vi "BRig_RT_panel_Laser1_v1,11.vi"(7 "input_setValues":bool, 9 "input_dataExp":u16[](array[numeric]), 11 "input_dataLC":u16[](array[numeric])) -> (1 "output_dataExp":u16[](array[numeric]), 3 "output_dataLC":u16[](array[numeric]))   [LabVIEW 2014]
panel:
  in  "LC_Sel_nRew2":u16
  in  "LC_Sel_nRew1":u16
  in  "LC_Cue2_nRew2":u16
  in  "LC_Cue2_nRew1":u16
  in  "LC_Cue_nRew2":u16
  in  "LC_Cue_nRew1":u16
  in  "LC_ENL2_nRew2":u16
  in  "LC_ENL2_nRew1":u16
  in  "LC_ENL_nRew2":u16
  in  "LC_ENL_nRew1":u16
  in  "LC_Cue2_PostR_Count":u16
  in  "LC_Cue2_PostR_delayOpt":bool
  in  "LC_Cue2_PostR_Probability":u16
  in  "LC_Cue2_PostR_Block":u16(slide) max=2 step=1 scale=0.0..2.0
  in  "LC_Cue2_PostR_OnOff":bool
  in  "LC_Cue2_PostR_Tdelay":u16
  in  "LC_ENL2_PostR_delayOpt":bool
  in  "LC_ENL2_PostR_Count":u16
  in  "LC_ENL2_PostR_Probability":u16 max=100 step=1
  in  "LC_ENL2_PostR_Block":u16(slide) max=2 step=1 scale=0.0..2.0
  in  "LC_ENL2_PostR_OnOff":bool
  in  "LC_ENL2_PostR_Tdelay":u16
  in  "LC_Cue2_PreR_Count":u16
  in  "LC_Cue2_First_Count":u16
  in  "LC_Cue2_PreR_delayOpt":bool
  in  "LC_ENL2_PreR_delayOpt":bool
  in  "LC_ENL2_PreR_Count":u16
  in  "LC_ENL2_First_Count":u16
  in  "LC_Cue2_First_delayOpt":bool
  in  "LC_ENL2_First_delayOpt":bool
  in  "LC_Cue2_PreR_Probability":u16
  in  "LC_Cue2_PreR_Block":u16(slide) max=2 step=1 scale=0.0..2.0
  in  "LC_Cue2_PreR_OnOff":bool
  in  "LC_Cue2_First_Probability":u16
  in  "LC_Cue2_First_Block":u16(slide) max=2 step=1 scale=0.0..2.0
  in  "LC_Cue2_First_OnOff":bool
  in  "LC_ENL2_PreR_Probability":u16 max=100 step=1
  in  "LC_ENL2_PreR_Block":u16(slide) max=2 step=1 scale=0.0..2.0
  in  "LC_ENL2_PreR_OnOff":bool
  in  "LC_ENL2_First_Probability":u16 max=100 step=1
  in  "LC_ENL2_First_Block":u16(slide) max=2 step=1 scale=0.0..2.0
  in  "LC_Cue2_PreR_Tdelay":u16
  in  "LC_ENL2_PreR_Tdelay":u16
  in  "LC_Cue2_First_Tdelay":u16
  in  "LC_ENL2_First_Tdelay":u16
  in  "LC_ENL2_First_OnOff":bool
  out "LaserPulseTrain":cluster{u16[], u16[]}(graph)
  in  "LED_baseline":bool
  in  "Laser_power_step":dbl
  in  "Laser_power_max":dbl
  in  "Laser_power_min":dbl
  in  "Laser_Tshutter":u16=2
  in  "Laser_Freq":u16=10
  in  "Laser_Tpeak":u16=2
  in  "Laser_T":u16
  in  "LC_Sel_PostR_Count":u16
  in  "LC_Sel_PostR_Probability":u16
  in  "LC_Sel_PostR_Block":u16(slide) max=2 step=1 scale=0.0..2.0
  in  "LC_Sel_PostR_OnOff":bool
  in  "LC_Sel_PostR_Tdelay":u16
  in  "LC_Cue_PostR_Count":u16
  in  "LC_Cue_PostR_delayOpt":bool
  in  "LC_Cue_PostR_Probability":u16
  in  "LC_Cue_PostR_Block":u16(slide) max=2 step=1 scale=0.0..2.0
  in  "LC_Cue_PostR_OnOff":bool
  in  "LC_Cue_PostR_Tdelay":u16
  in  "LC_ENL_PostR_delayOpt":bool
  in  "LC_ENL_PostR_Count":u16
  in  "LC_ENL_PostR_Probability":u16 max=100 step=1
  in  "LC_ENL_PostR_Block":u16(slide) max=2 step=1 scale=0.0..2.0
  in  "LC_ENL_PostR_OnOff":bool
  in  "LC_ENL_PostR_Tdelay":u16
  in  "LC_Sel_PreR_Count":u16
  in  "LC_Sel_First_Count":u16
  in  "LC_Sel_PreR_Probability":u16
  in  "LC_Sel_PreR_Block":u16(slide) max=2 step=1 scale=0.0..2.0
  in  "LC_Sel_PreR_OnOff":bool
  in  "LC_Sel_First_Probability":u16
  in  "LC_Sel_First_Block":u16(slide) max=2 step=1 scale=0.0..2.0
  in  "LC_Sel_First_OnOff":bool
  in  "LC_Sel_PreR_Tdelay":u16
  in  "LC_Sel_First_Tdelay":u16
  in  "LC_Cue_PreR_Count":u16
  in  "LC_Cue_First_Count":u16
  in  "LC_Cue_PreR_delayOpt":bool
  in  "LC_ENL_PreR_delayOpt":bool
  in  "LC_ENL_PreR_Count":u16
  in  "LC_ENL_First_Count":u16
  in  "LC_Cue_First_delayOpt":bool
  in  "LC_ENL_First_delayOpt":bool
  in  "LC_Wrong_Probability":u16
  in  "LC_Wrong_Trial":u16(slide) max=2 step=1 scale=0.0..2.0
  in  "LC_Wrong_Block":u16(slide) max=2 step=1 scale=0.0..2.0
  in  "LC_Wrong_OnOff":bool
  in  "LC_Reward_Probability":u16
  in  "LC_Reward_Trial":u16(slide) max=2 step=1 scale=0.0..2.0
  in  "LC_Reward_Block":u16(slide) max=2 step=1 scale=0.0..2.0
  in  "LC_Reward_OnOff":bool
  in  "LC_Cue_PreR_Probability":u16
  in  "LC_Cue_PreR_Block":u16(slide) max=2 step=1 scale=0.0..2.0
  in  "LC_Cue_PreR_OnOff":bool
  in  "LC_Cue_First_Probability":u16
  in  "LC_Cue_First_Block":u16(slide) max=2 step=1 scale=0.0..2.0
  in  "LC_Cue_First_OnOff":bool
  in  "LC_ENL_PreR_Probability":u16 max=100 step=1
  in  "LC_ENL_PreR_Block":u16(slide) max=2 step=1 scale=0.0..2.0
  in  "LC_ENL_PreR_OnOff":bool
  in  "LC_ENL_First_Probability":u16 max=100 step=1
  in  "LC_ENL_First_Block":u16(slide) max=2 step=1 scale=0.0..2.0
  in  "LC_Wrong_Tdelay":u16
  in  "LC_Cue_PreR_Tdelay":u16
  in  "LC_ENL_PreR_Tdelay":u16
  in  "LC_Reward_Tdelay":u16
  in  "LC_Cue_First_Tdelay":u16
  in  "LC_ENL_First_Tdelay":u16
  in  "LC_ENL_First_OnOff":bool
  # "Laser1 Control\n                               On/Off      Block        Probability [%]   Delay [ms]                              Count"
  # "On/Off      Block        Probability [%]   Delay [ms]                              Count"
  # "Enforced\nNonLick"
  # "Enforced\nNonLick\n     2"
  # "from end"
  # "from end"
  # "First\nTrial"
  # "First\nTrial"
  # "from start"
  # "from start"
  # "from end"
  # "from end"
  # "PreReward\nTrials"
  # "PreReward\nTrials"
  # "from start"
  # "from start"
  # "from end"
  # "from end"
  # "PostReward\nTrials"
  # "PostReward\nTrials"
  # "from start"
  # "from start"
  # "PostReward Option - Trigger after [X1] or [X2] reward\n                                        (0 = ignore this option)"
  # "PostReward Option - Trigger after [X1] or [X2] reward\n                                        (0 = ignore this option)"
  # "Cue"
  # "Cue\n  2"
  # "from end"
  # "from end"
  # "First\nTrial"
  # "First\nTrial"
  # "from start"
  # "from start"
  # "from end"
  # "from end"
  # "PreReward\nTrials"
  # "PreReward\nTrials"
  # "from start"
  # "from start"
  # "from end"
  # "from end"
  # "PostReward\nTrials"
  # "PostReward\nTrials"
  # "from start"
  # "from start"
  # "PostReward Option - Trigger after [X1] or [X2] reward\n                                        (0 = ignore this option)"
  # "PostReward Option - Trigger after [X1] or [X2] reward\n                                        (0 = ignore this option)"
  # "Selection"
  # "from start"
  # "First\nTrial"
  # "from start"
  # "PreReward\nTrials"
  # "from start"
  # "PostReward\nTrials"
  # "PostReward Option - Trigger after [X1] or [X2] reward\n                                        (0 = ignore this option)"
  # "Laser1 Parameters"
  # "Laser1 Response\n           On/Off      Block           Trial     Probability %  Delay [ms]"
  # "Frequency\n[Hz]"
  # "Selection\nReward"
  # "Timing [ms]\n Duration     Peak Width   Shutter"
  # "Selection\nWrong"
  # "Laser Power [V]\nMin          Max              Step"
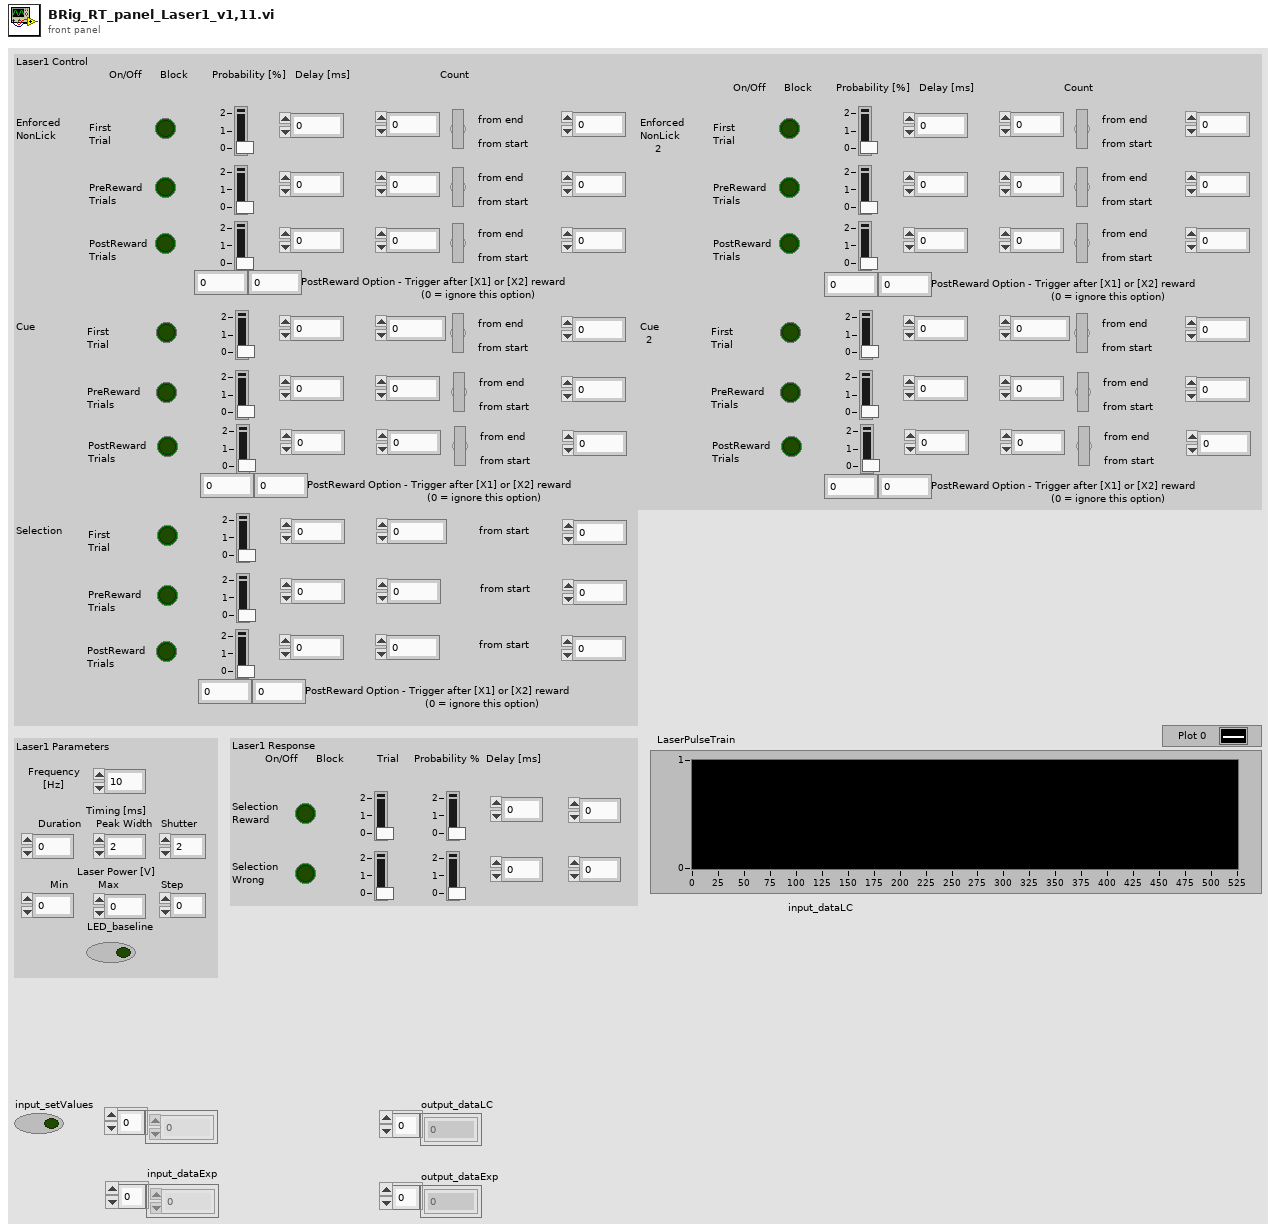
[diagram p1: front panel]
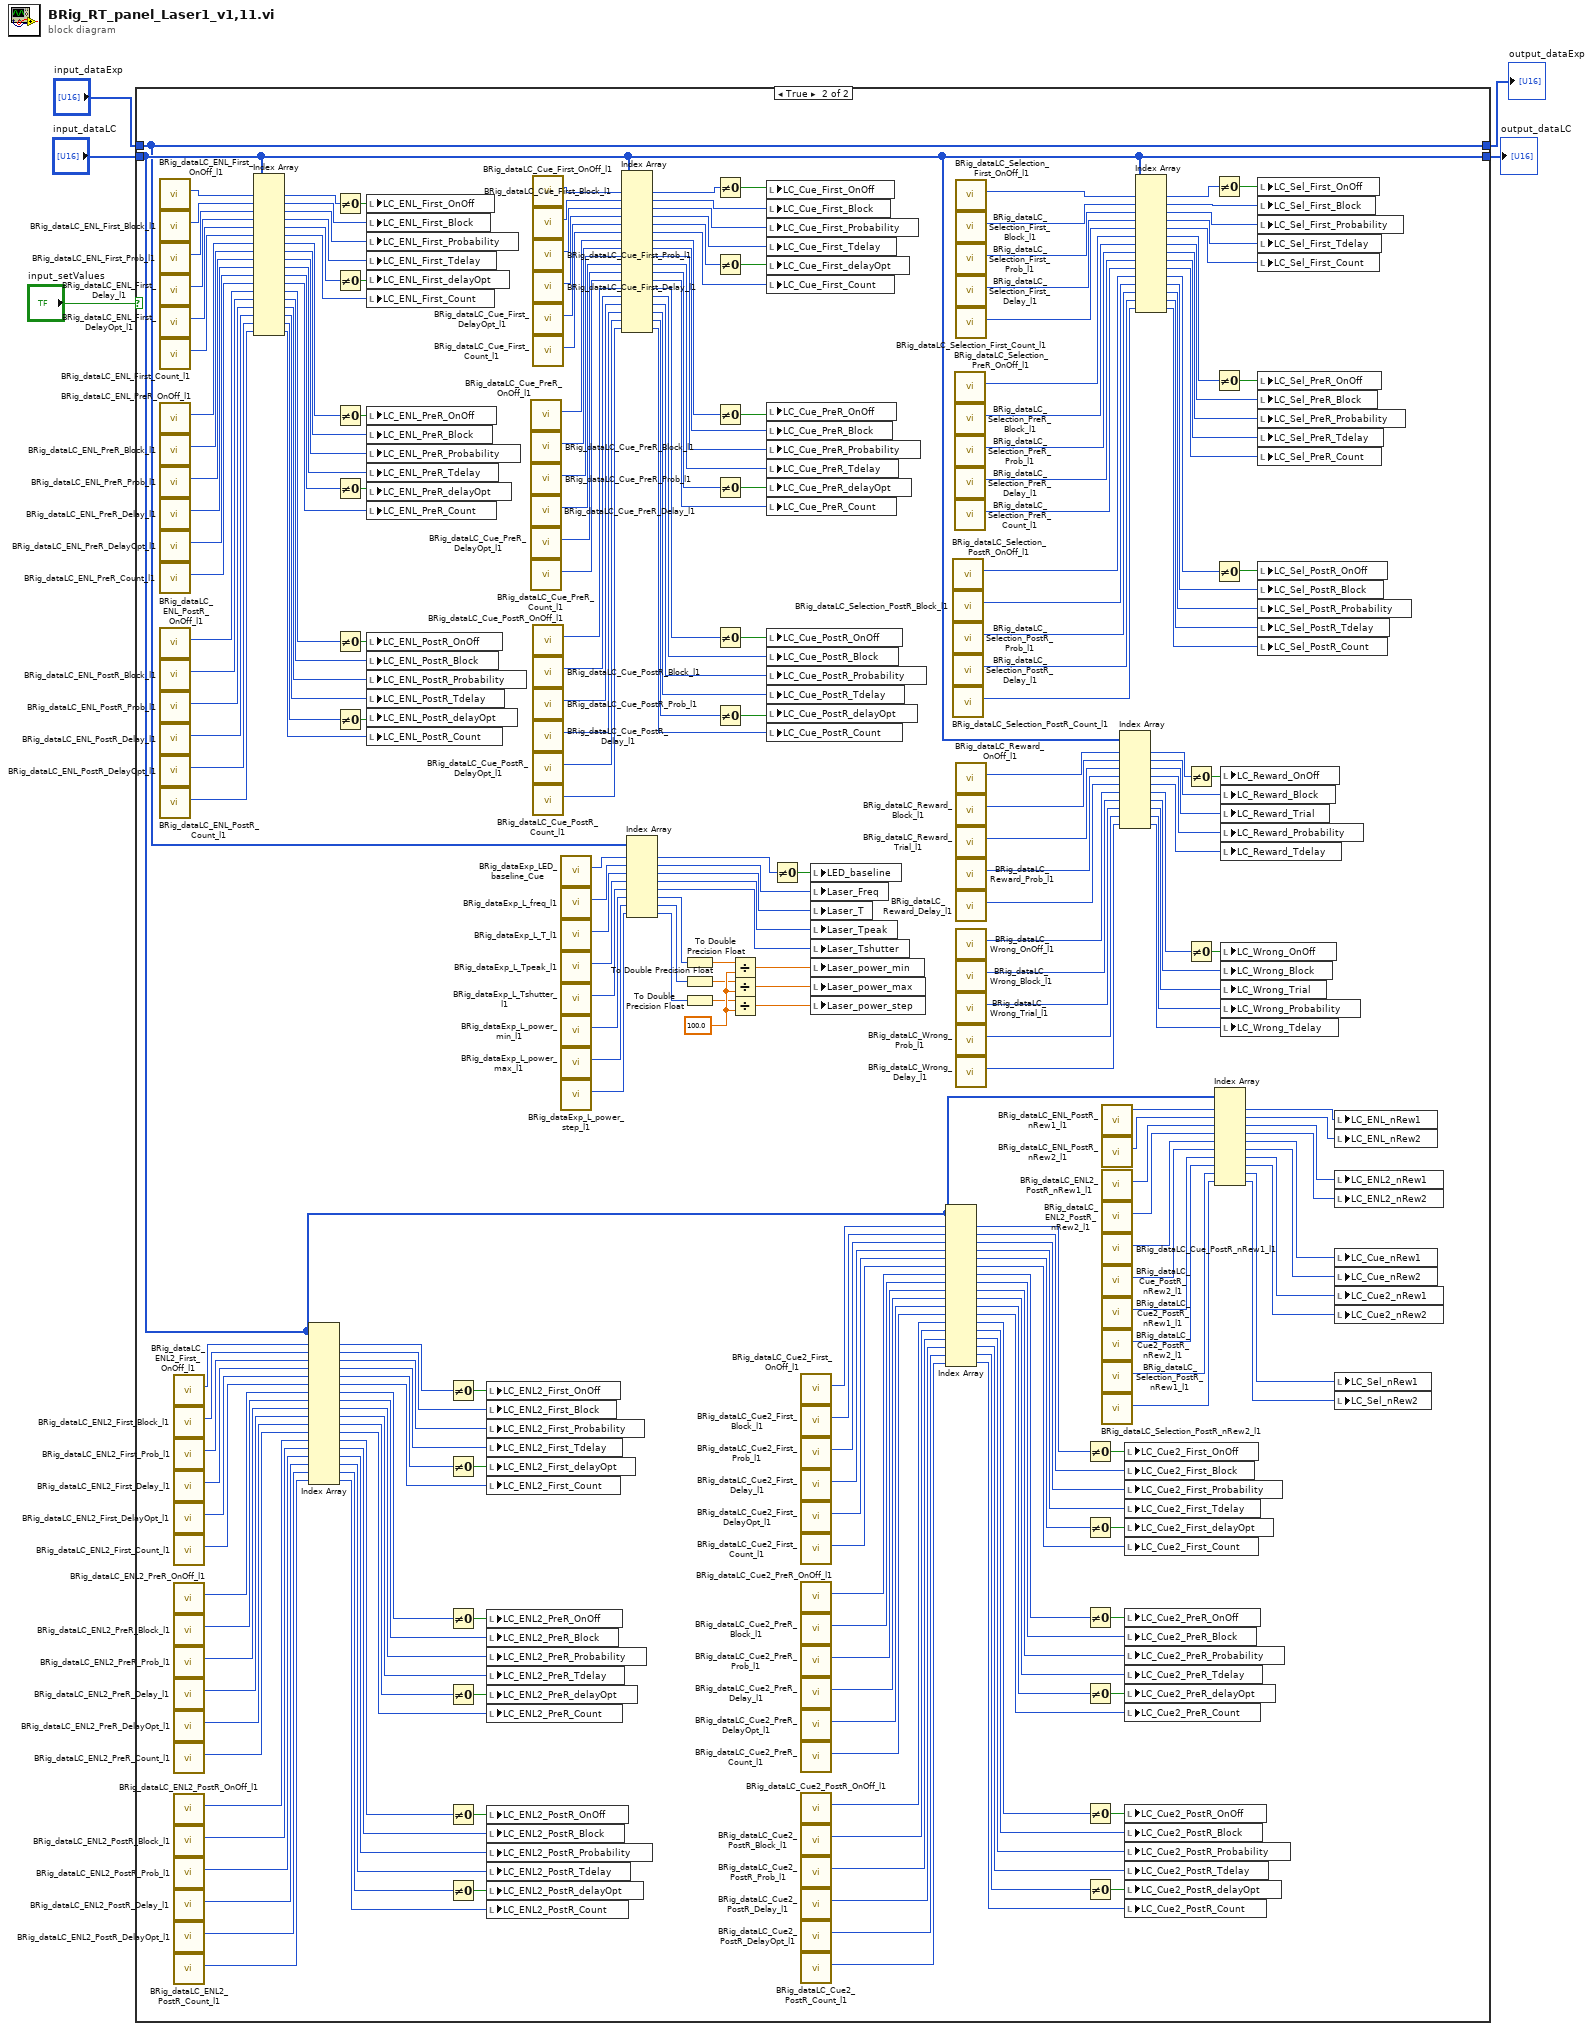
[diagram p0: block diagram]
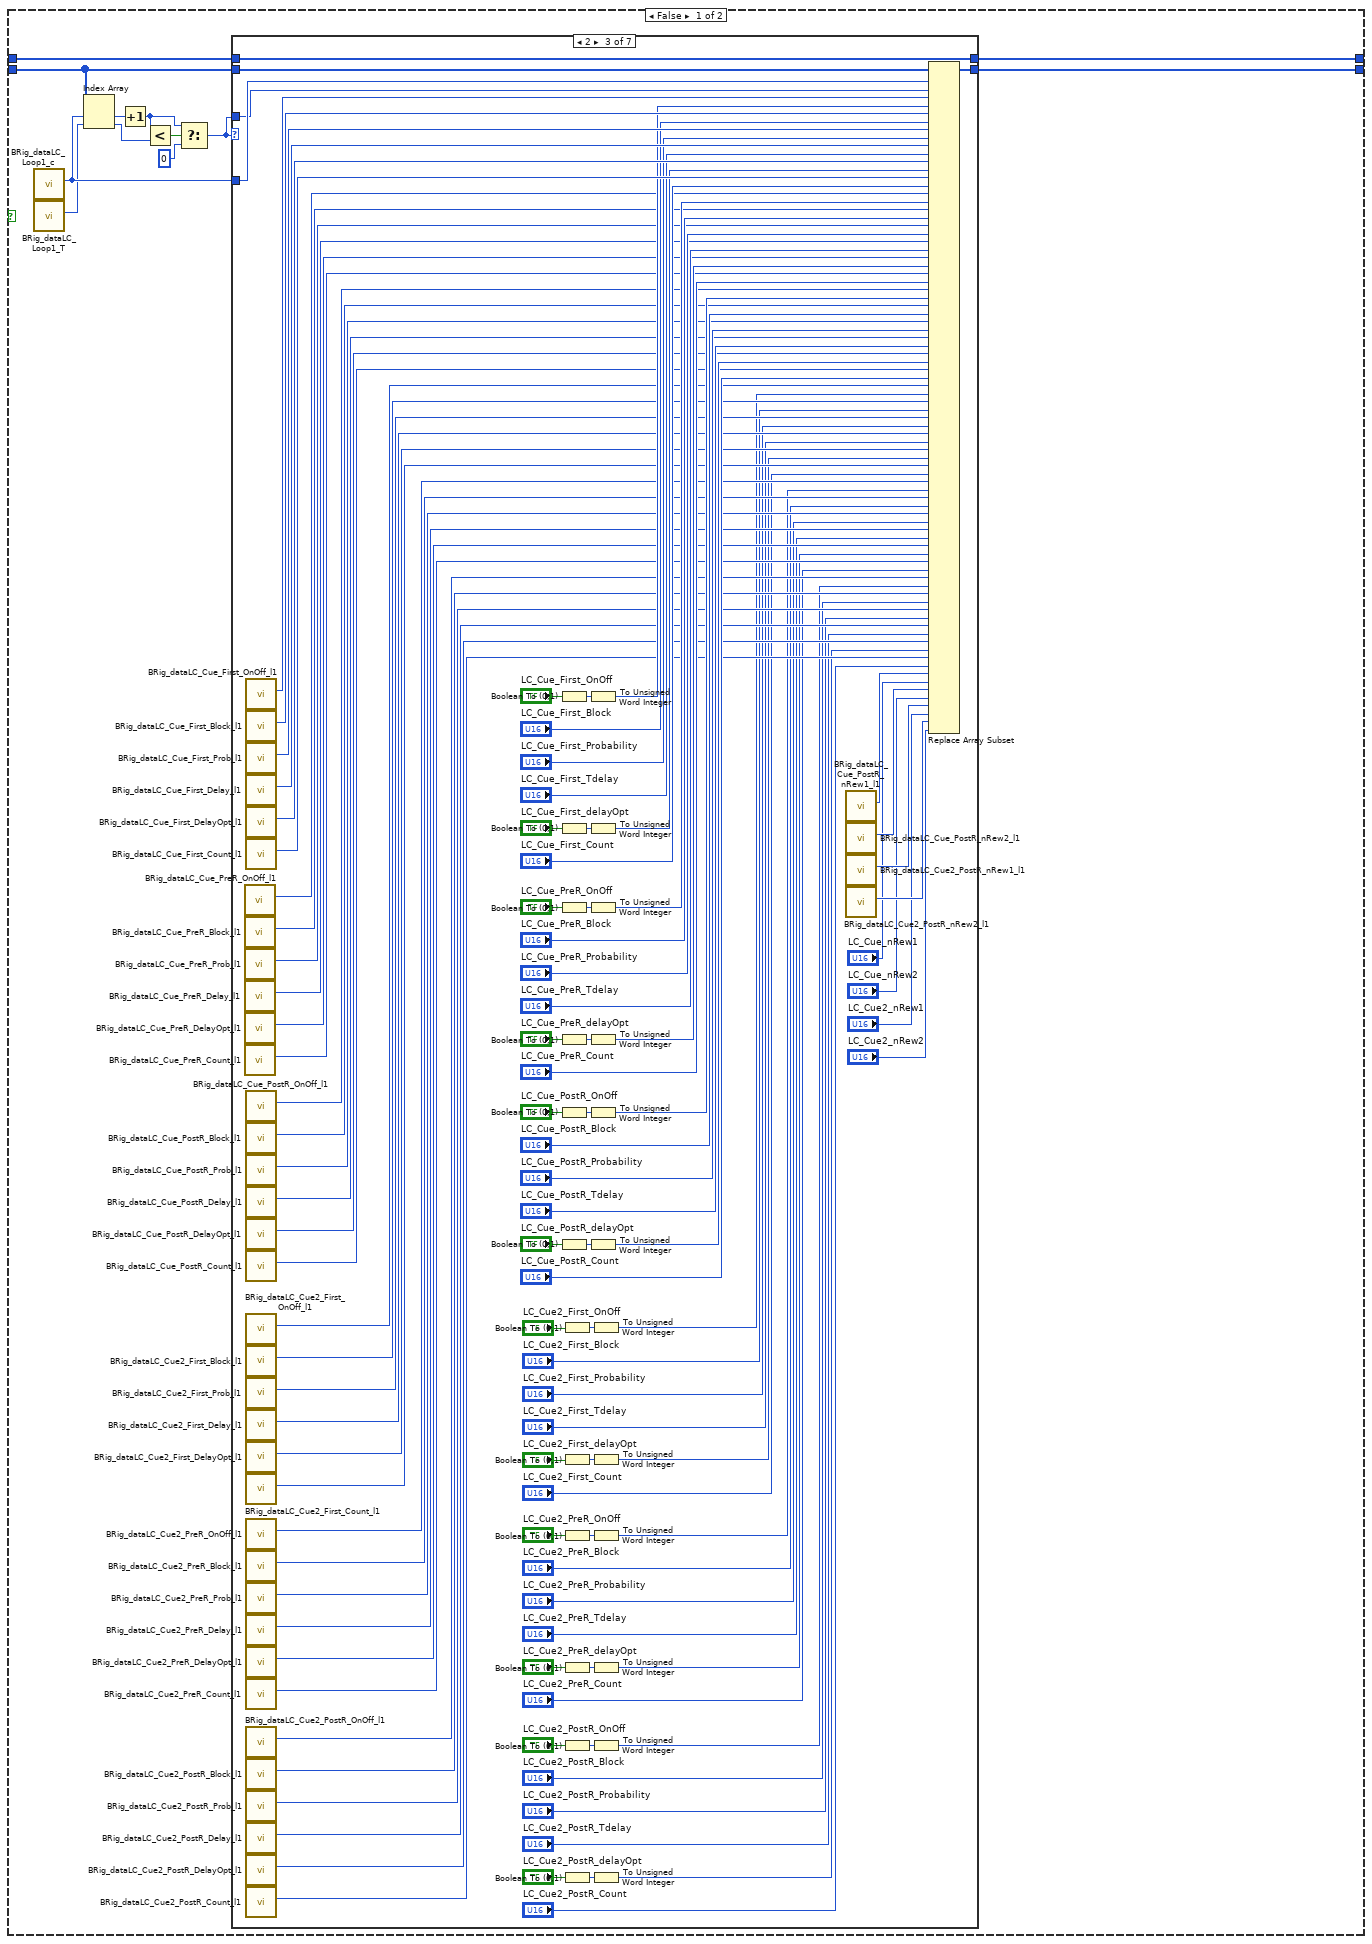
[diagram p2: hidden frame]
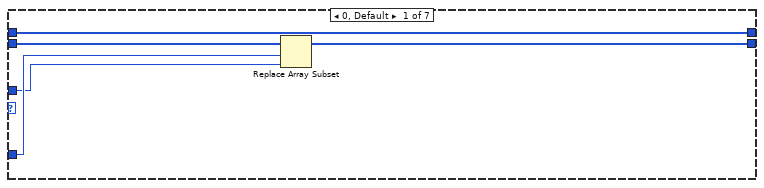
[diagram p3: hidden frame]
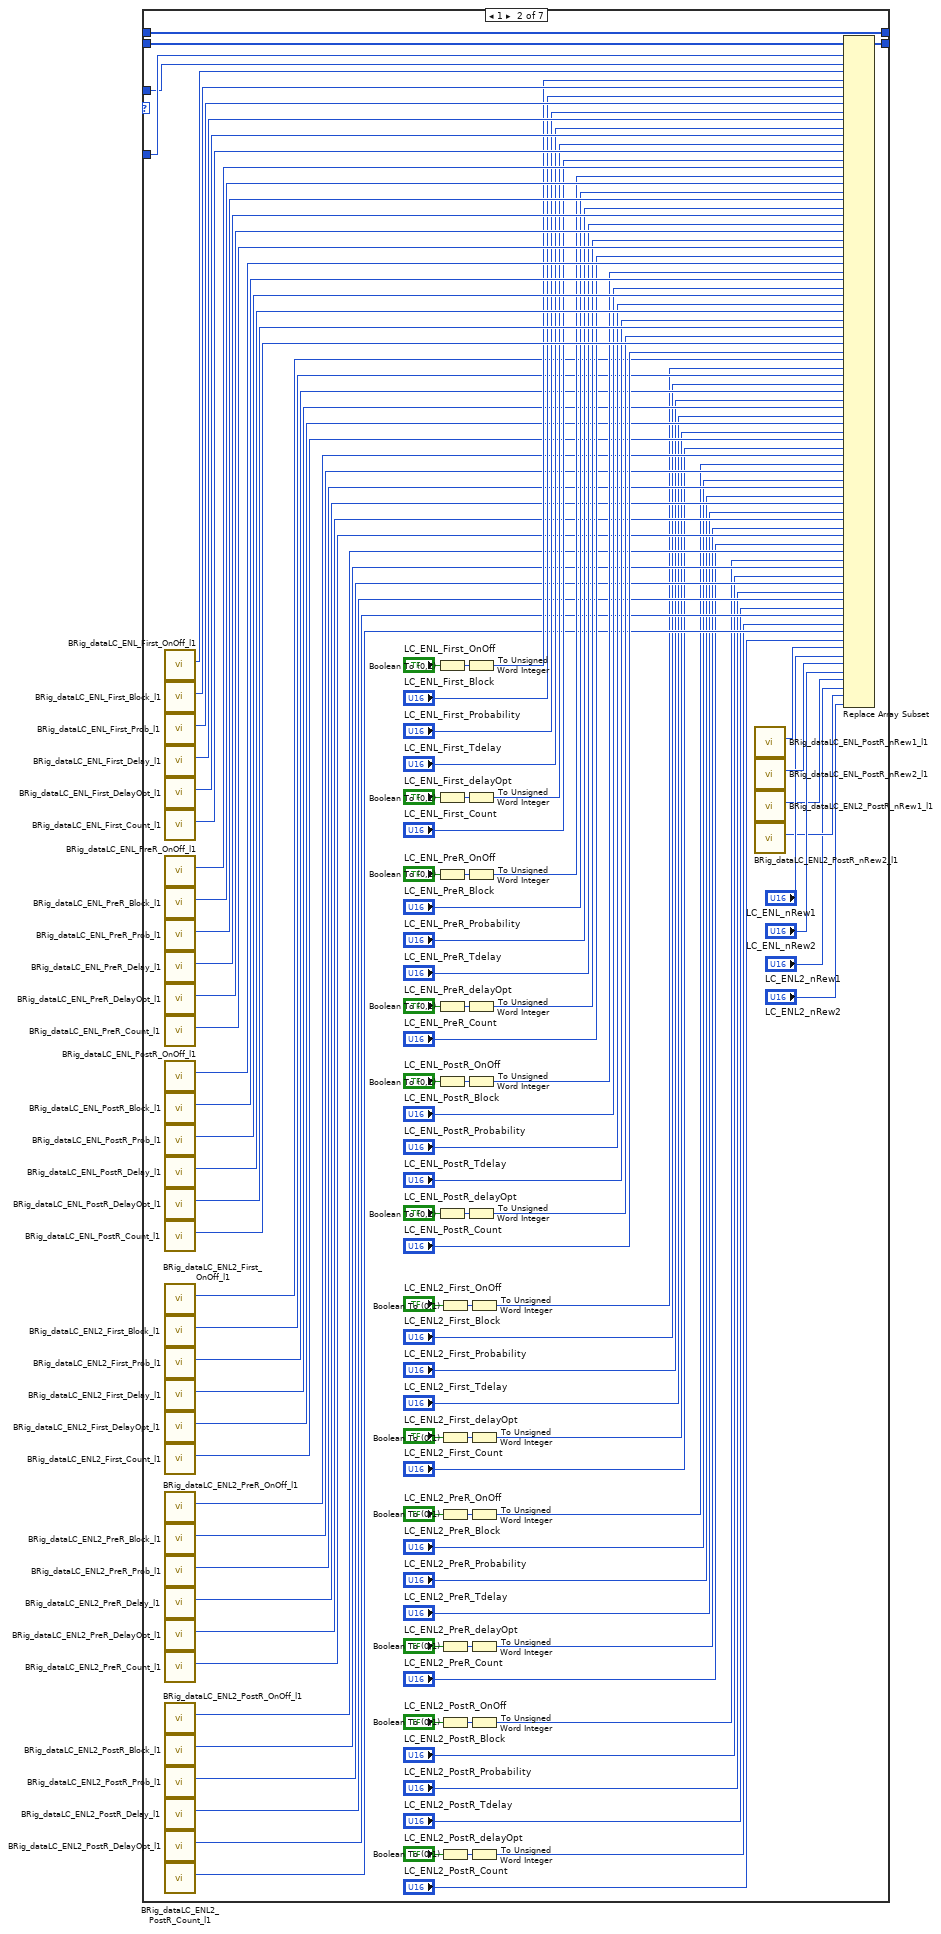
[diagram p4: hidden frame]
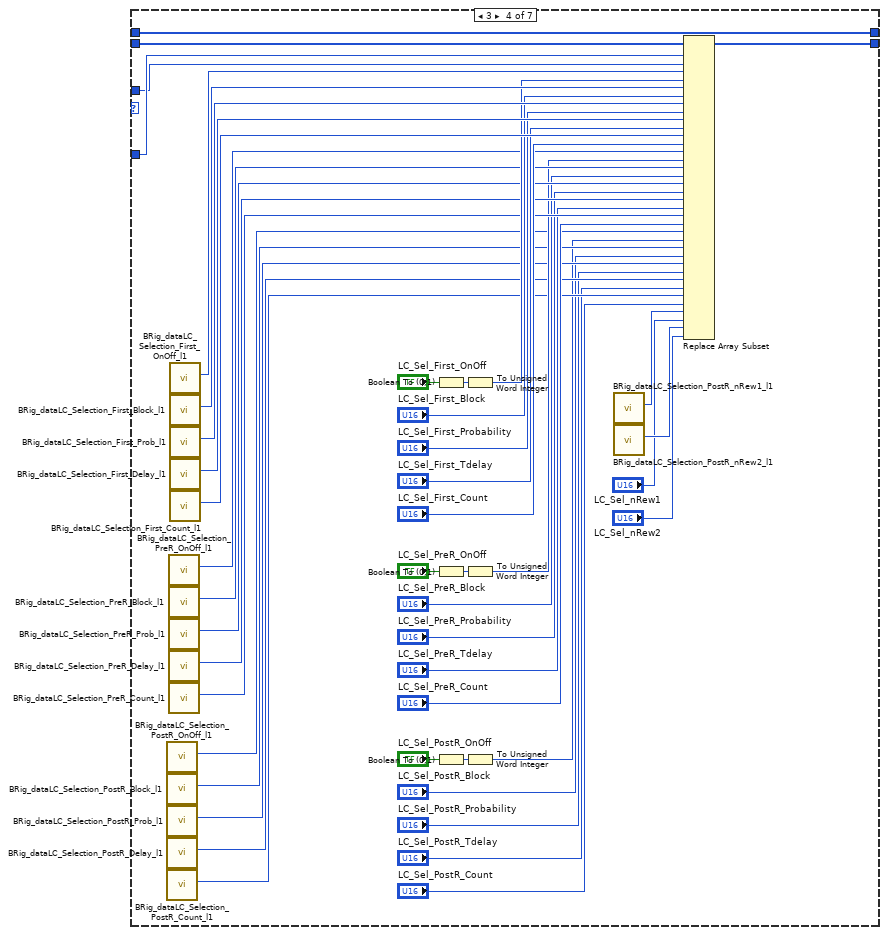
[diagram p5: hidden frame]
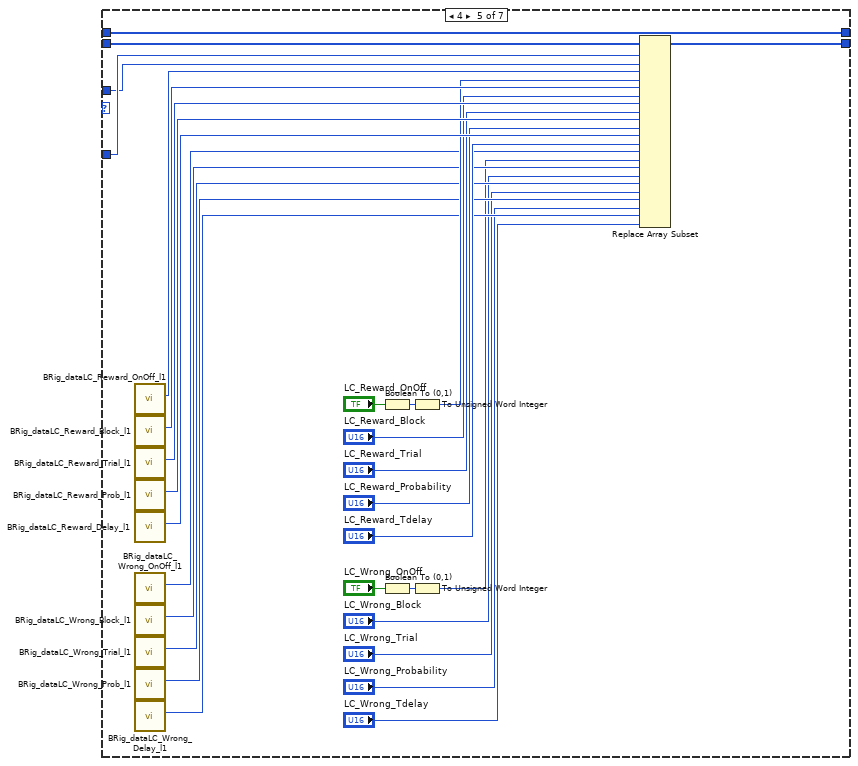
[diagram p6: hidden frame]
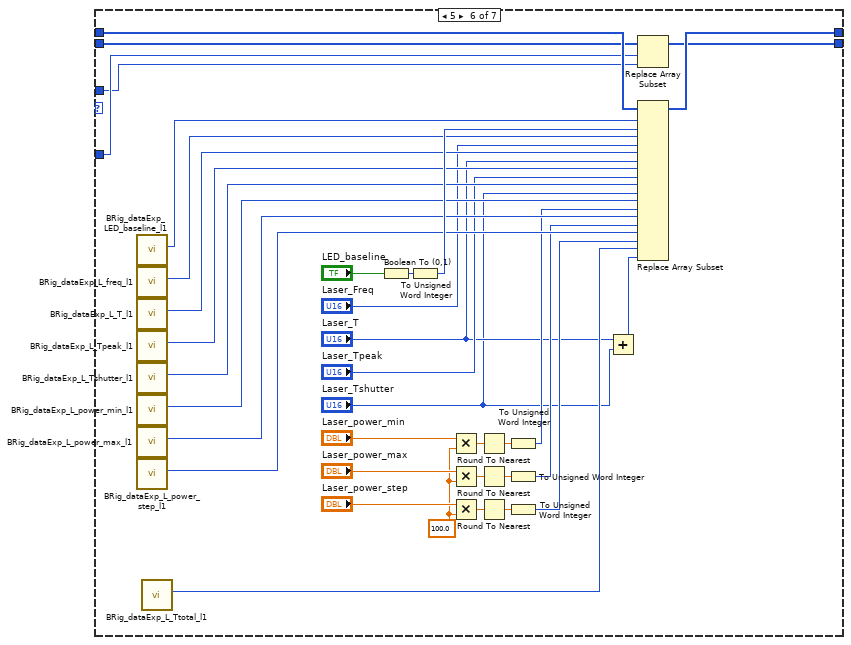
[diagram p7: hidden frame]
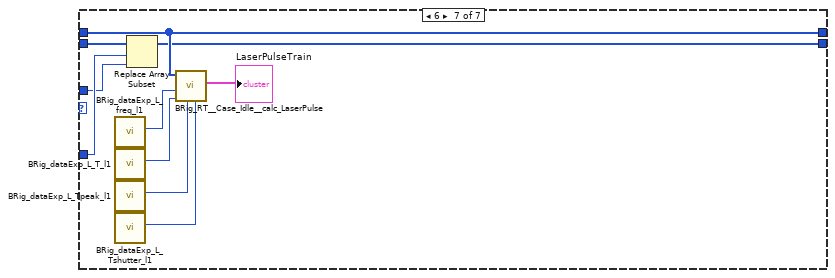
[diagram p8: hidden frame]
diagram:
  n1 = case shown="True" "input_setValues" {
    tunnel: "input_dataLC" -> [w17 w378]
    tunnel: [w11 w378] -> w4
    tunnel: "input_dataExp" -> [w7 w377]
    tunnel: [w6 w377] -> w1
    frame False {
      n2 = call "BRig_dataLC_Loop1_c.vi"() -> ("output_Loop1_c"=w10:i32)  [unwired: 11 in]
      n3 = call "BRig_dataLC_Loop1_T.vi"() -> ("output_Loop1_T"=w9:i32)  [unwired: 11 in]
      n4 = Index Array(array=w17, index #1=w10, index #2=w9) -> (element #1=w16:u16, element #2=w15:u16)
      n5 = Increment(x=w16) -> (x+1=w12:u16)
      n6 = Less?(x=w12, y=w15) -> (x < y?=w14:bool)
      n7 = Select(t=w12, s=w14, f=u16 0) -> (s? t:f=w8:u16)
      n8 = case shown="2" w8 {
        tunnel: w17 -> [w22 w131 w240 w285 w314 w319 w358]
        tunnel: w10 -> [w20 w81 w202 w247 w288 w317 w356]
        tunnel: w8 -> [w19 w80 w201 w246 w287 w316 w355]
        tunnel: [w21 w124 w239 w284 w313 w318 w357] -> w11
        tunnel: w7 -> [w18 w79 w188 w245 w286 w321 w360]
        tunnel: [w18 w79 w188 w245 w286 w320 w360] -> w6
        frame 0, Default {
          n9 = Replace Array Subset(array=w22, new element=w19, index=w20) -> (w21:u16[])
        }
        frame 1 {
          n10 = call "BRig_dataLC_ENL_First_OnOff_l1.vi"() -> ("output_ENL_First_OnOff"=w130:i32)  [unwired: 11 in]
          n11 = call "BRig_dataLC_ENL_First_Block_l1.vi"() -> ("output_ENL_First_Block"=w129:i32)  [unwired: 11 in]
          n12 = call "BRig_dataLC_ENL_First_Prob_l1.vi"() -> ("output_ENL_First_Prob"=w128:i32)  [unwired: 11 in]
          n13 = call "BRig_dataLC_ENL_First_Delay_l1.vi"() -> ("output_ENL_First_Delay"=w127:i32)  [unwired: 11 in]
          n14 = call "BRig_dataLC_ENL_First_DelayOpt_l1.vi"() -> ("output_ENL_First_DelayOpt"=w126:i32)  [unwired: 11 in]
          n15 = call "BRig_dataLC_ENL_First_Count_l1.vi"() -> ("output_ENL_First_Count"=w125:i32)  [unwired: 11 in]
          n16 = call "BRig_dataLC_ENL_PreR_OnOff_l1.vi"() -> ("output_ENL_PreR_OnOff"=w123:i32)  [unwired: 11 in]
          n17 = call "BRig_dataLC_ENL_PreR_Block_l1.vi"() -> ("output_ENL_PreR_Block"=w122:i32)  [unwired: 11 in]
          n18 = call "BRig_dataLC_ENL_PreR_Prob_l1.vi"() -> ("output_ENL_PreR_Prob"=w121:i32)  [unwired: 11 in]
          n19 = call "BRig_dataLC_ENL_PreR_Delay_l1.vi"() -> ("output_ENL_PreR_Delay"=w120:i32)  [unwired: 11 in]
          n20 = call "BRig_dataLC_ENL_PreR_DelayOpt_l1.vi"() -> ("output_ENL_PreR_DelayOpt"=w119:i32)  [unwired: 11 in]
          n21 = call "BRig_dataLC_ENL_PreR_Count_l1.vi"() -> ("output_ENL_PreR_Count"=w118:i32)  [unwired: 11 in]
          n22 = call "BRig_dataLC_ENL_PostR_OnOff_l1.vi"() -> ("output_ENL_PostR_OnOff"=w117:i32)  [unwired: 11 in]
          n23 = call "BRig_dataLC_ENL_PostR_Block_l1.vi"() -> ("output_ENL_PostR_Block"=w116:i32)  [unwired: 11 in]
          n24 = call "BRig_dataLC_ENL_PostR_Prob_l1.vi"() -> ("output_ENL_PostR_Prob"=w115:i32)  [unwired: 11 in]
          n25 = call "BRig_dataLC_ENL_PostR_Delay_l1.vi"() -> ("output_ENL_PostR_Delay"=w114:i32)  [unwired: 11 in]
          n26 = call "BRig_dataLC_ENL_PostR_DelayOpt_l1.vi"() -> ("output_ENL_PostR_DelayOpt"=w113:i32)  [unwired: 11 in]
          n27 = call "BRig_dataLC_ENL_PostR_Count_l1.vi"() -> ("output_ENL_PostR_Count"=w112:i32)  [unwired: 11 in]
          n28 = call "BRig_dataLC_ENL2_First_OnOff_l1.vi"() -> ("output_ENL2_First_OnOff"=w78:i32)  [unwired: 11 in]
          n29 = call "BRig_dataLC_ENL2_First_Block_l1.vi"() -> ("output_ENL2_First_Block"=w77:i32)  [unwired: 11 in]
          n30 = call "BRig_dataLC_ENL2_First_Prob_l1.vi"() -> ("output_ENL2_First_Prob"=w76:i32)  [unwired: 11 in]
          n31 = call "BRig_dataLC_ENL2_First_Delay_l1.vi"() -> ("output_ENL2_First_Delay"=w75:i32)  [unwired: 11 in]
          n32 = call "BRig_dataLC_ENL2_First_DelayOpt_l1.vi"() -> ("output_ENL2_First_DelayOpt"=w74:i32)  [unwired: 11 in]
          n33 = call "BRig_dataLC_ENL2_First_Count_l1.vi"() -> ("output_ENL2_First_Count"=w73:i32)  [unwired: 11 in]
          n34 = call "BRig_dataLC_ENL2_PreR_OnOff_l1.vi"() -> ("output_ENL2_PreR_OnOff"=w72:i32)  [unwired: 11 in]
          n35 = call "BRig_dataLC_ENL2_PreR_Block_l1.vi"() -> ("output_ENL2_PreR_Block"=w71:i32)  [unwired: 11 in]
          n36 = call "BRig_dataLC_ENL2_PreR_Prob_l1.vi"() -> ("output_ENL2_PreR_Prob"=w70:i32)  [unwired: 11 in]
          n37 = call "BRig_dataLC_ENL2_PreR_Delay_l1.vi"() -> ("output_ENL2_PreR_Delay"=w69:i32)  [unwired: 11 in]
          n38 = call "BRig_dataLC_ENL2_PreR_DelayOpt_l1.vi"() -> ("output_ENL2_PreR_DelayOpt"=w68:i32)  [unwired: 11 in]
          n39 = call "BRig_dataLC_ENL2_PreR_Count_l1.vi"() -> ("output_ENL2_PreR_Count"=w67:i32)  [unwired: 11 in]
          n40 = call "BRig_dataLC_ENL2_PostR_OnOff_l1.vi"() -> ("output_ENL2_PostR_OnOff"=w66:i32)  [unwired: 11 in]
          n41 = call "BRig_dataLC_ENL2_PostR_Block_l1.vi"() -> ("output_ENL2_PostR_Block"=w65:i32)  [unwired: 11 in]
          n42 = call "BRig_dataLC_ENL2_PostR_Prob_l1.vi"() -> ("output_ENL2_PostR_Prob"=w64:i32)  [unwired: 11 in]
          n43 = call "BRig_dataLC_ENL2_PostR_Delay_l1.vi"() -> ("output_ENL2_PostR_Delay"=w63:i32)  [unwired: 11 in]
          n44 = call "BRig_dataLC_ENL2_PostR_DelayOpt_l1.vi"() -> ("output_ENL2_PostR_DelayOpt"=w62:i32)  [unwired: 11 in]
          n45 = call "BRig_dataLC_ENL2_PostR_Count_l1.vi"() -> ("output_ENL2_PostR_Count"=w61:i32)  [unwired: 11 in]
          n46 = Boolean To (0,1)(Boolean="LC_ENL_First_OnOff") -> (0, 1=w110:i16)
          n47 = Boolean To (0,1)(Boolean="LC_ENL_First_delayOpt") -> (0, 1=w109:i16)
          n48 = Boolean To (0,1)(Boolean="LC_ENL_PreR_OnOff") -> (0, 1=w107:i16)
          n49 = Boolean To (0,1)(Boolean="LC_ENL_PreR_delayOpt") -> (0, 1=w105:i16)
          n50 = Boolean To (0,1)(Boolean="LC_ENL_PostR_OnOff") -> (0, 1=w103:i16)
          n51 = Boolean To (0,1)(Boolean="LC_ENL_PostR_delayOpt") -> (0, 1=w101:i16)
          n52 = Boolean To (0,1)(Boolean="LC_ENL2_First_OnOff") -> (0, 1=w51:i16)
          n53 = Boolean To (0,1)(Boolean="LC_ENL2_First_delayOpt") -> (0, 1=w50:i16)
          n54 = Boolean To (0,1)(Boolean="LC_ENL2_PreR_OnOff") -> (0, 1=w49:i16)
          n55 = Boolean To (0,1)(Boolean="LC_ENL2_PreR_delayOpt") -> (0, 1=w47:i16)
          n56 = Boolean To (0,1)(Boolean="LC_ENL2_PostR_OnOff") -> (0, 1=w39:i16)
          n57 = Boolean To (0,1)(Boolean="LC_ENL2_PostR_delayOpt") -> (0, 1=w37:i16)
          n58 = To Unsigned Word Integer(number=w110) -> (unsigned 16bit integer=w99:u16)
          n59 = To Unsigned Word Integer(number=w109) -> (unsigned 16bit integer=w95:u16)
          n60 = To Unsigned Word Integer(number=w107) -> (unsigned 16bit integer=w93:u16)
          n61 = To Unsigned Word Integer(number=w105) -> (unsigned 16bit integer=w89:u16)
          n62 = To Unsigned Word Integer(number=w103) -> (unsigned 16bit integer=w87:u16)
          n63 = To Unsigned Word Integer(number=w101) -> (unsigned 16bit integer=w83:u16)
          n64 = To Unsigned Word Integer(number=w51) -> (unsigned 16bit integer=w58:u16)
          n65 = To Unsigned Word Integer(number=w50) -> (unsigned 16bit integer=w54:u16)
          n66 = To Unsigned Word Integer(number=w49) -> (unsigned 16bit integer=w52:u16)
          n67 = To Unsigned Word Integer(number=w47) -> (unsigned 16bit integer=w42:u16)
          n68 = To Unsigned Word Integer(number=w39) -> (unsigned 16bit integer=w40:u16)
          n69 = To Unsigned Word Integer(number=w37) -> (unsigned 16bit integer=w32:u16)
          n70 = call "BRig_dataLC_ENL_PostR_nRew1_l1.vi"() -> ("output_ENL_PostR_nRew1_l1"=w30:i32)  [unwired: 11 in]
          n71 = call "BRig_dataLC_ENL_PostR_nRew2_l1.vi"() -> ("output_ENL_PostR_nRew2_l1"=w29:i32)  [unwired: 11 in]
          n72 = call "BRig_dataLC_ENL2_PostR_nRew1_l1.vi"() -> ("output_ENL2_PostR_nRew1_l1"=w26:i32)  [unwired: 11 in]
          n73 = call "BRig_dataLC_ENL2_PostR_nRew2_l1.vi"() -> ("output_ENL2_PostR_nRew2_l1"=w25:i32)  [unwired: 11 in]
          n74 = Replace Array Subset(array=w131, new element #1=w80, index #1=w81, new element #2=w99, index #2=w130, new element #3="LC_ENL_First_Block", index #3=w129, new element #4="LC_ENL_First_Probability", index #4=w128, new element #5="LC_ENL_First_Tdelay", index #5=w127, new element #6=w95, index #6=w126, new element #7="LC_ENL_First_Count", index #7=w125, new element #8=w93, index #8=w123, new element #9="LC_ENL_PreR_Block", index #9=w122, new element #10="LC_ENL_PreR_Probability", index #10=w121, new element #11="LC_ENL_PreR_Tdelay", index #11=w120, new element #12=w89, index #12=w119, new element #13="LC_ENL_PreR_Count", index #13=w118, new element #14=w87, index #14=w117, new element #15="LC_ENL_PostR_Block", index #15=w116, new element #16="LC_ENL_PostR_Probability", index #16=w115, new element #17="LC_ENL_PostR_Tdelay", index #17=w114, new element #18=w83, index #18=w113, new element #19="LC_ENL_PostR_Count", index #19=w112, new element #20=w58, index #20=w78, new element #21="LC_ENL2_First_Block", index #21=w77, new element #22="LC_ENL2_First_Probability", index #22=w76, new element #23="LC_ENL2_First_Tdelay", index #23=w75, new element #24=w54, index #24=w74, new element #25="LC_ENL2_First_Count", index #25=w73, new element #26=w52, index #26=w72, new element #27="LC_ENL2_PreR_Block", index #27=w71, new element #28="LC_ENL2_PreR_Probability", index #28=w70, new element #29="LC_ENL2_PreR_Tdelay", index #29=w69, new element #30=w42, index #30=w68, new element #31="LC_ENL2_PreR_Count", index #31=w67, new element #32=w40, index #32=w66, new element #33="LC_ENL2_PostR_Block", index #33=w65, new element #34="LC_ENL2_PostR_Probability", index #34=w64, new element #35="LC_ENL2_PostR_Tdelay", index #35=w63, new element #36=w32, index #36=w62, new element #37="LC_ENL2_PostR_Count", index #37=w61, new element #38="LC_ENL_nRew1", index #38=w30, new element #39="LC_ENL_nRew2", index #39=w29, new element #40="LC_ENL2_nRew1", index #40=w26, new element #41="LC_ENL2_nRew2", index #41=w25) -> (w124:u16[])
        }
        frame 2 {
          n75 = call "BRig_dataLC_Cue_PreR_OnOff_l1.vi"() -> ("output_Cue_PreR_OnOff"=w198:i32)  [unwired: 11 in]
          n76 = call "BRig_dataLC_Cue_PreR_Block_l1.vi"() -> ("output_Cue_PreR_Block"=w197:i32)  [unwired: 11 in]
          n77 = call "BRig_dataLC_Cue_PreR_Prob_l1.vi"() -> ("output_Cue_PreR_Prob"=w196:i32)  [unwired: 11 in]
          n78 = call "BRig_dataLC_Cue_PreR_Delay_l1.vi"() -> ("output_Cue_PreR_Delay"=w195:i32)  [unwired: 11 in]
          n79 = call "BRig_dataLC_Cue_PreR_DelayOpt_l1.vi"() -> ("output_Cue_PreR_DelayOpt"=w194:i32)  [unwired: 11 in]
          n80 = call "BRig_dataLC_Cue_PreR_Count_l1.vi"() -> ("output_Cue_PreR_Count"=w199:i32)  [unwired: 11 in]
          n81 = call "BRig_dataLC_Cue_First_OnOff_l1.vi"() -> ("output_Cue_First_OnOff"=w238:i32)  [unwired: 11 in]
          n82 = call "BRig_dataLC_Cue_First_Block_l1.vi"() -> ("output_Cue_First_Block"=w237:i32)  [unwired: 11 in]
          n83 = call "BRig_dataLC_Cue_First_Prob_l1.vi"() -> ("output_Cue_First_Prob"=w236:i32)  [unwired: 11 in]
          n84 = call "BRig_dataLC_Cue_First_Delay_l1.vi"() -> ("output_Cue_First_Delay"=w235:i32)  [unwired: 11 in]
          n85 = call "BRig_dataLC_Cue_First_DelayOpt_l1.vi"() -> ("output_Cue_First_DelayOpt"=w234:i32)  [unwired: 11 in]
          n86 = call "BRig_dataLC_Cue_First_Count_l1.vi"() -> ("output_Cue_First_Count"=w233:i32)  [unwired: 11 in]
          n87 = call "BRig_dataLC_Cue_PostR_OnOff_l1.vi"() -> ("output_Cue_PostR_OnOff"=w200:i32)  [unwired: 11 in]
          n88 = call "BRig_dataLC_Cue_PostR_Block_l1.vi"() -> ("output_Cue_PostR_Block"=w193:i32)  [unwired: 11 in]
          n89 = call "BRig_dataLC_Cue_PostR_Prob_l1.vi"() -> ("output_Cue_PostR_Prob"=w192:i32)  [unwired: 11 in]
          n90 = call "BRig_dataLC_Cue_PostR_Delay_l1.vi"() -> ("output_Cue_PostR_Delay"=w191:i32)  [unwired: 11 in]
          n91 = call "BRig_dataLC_Cue_PostR_DelayOpt_l1.vi"() -> ("output_Cue_PostR_DelayOpt"=w190:i32)  [unwired: 11 in]
          n92 = call "BRig_dataLC_Cue_PostR_Count_l1.vi"() -> ("output_Cue_PostR_Count"=w189:i32)  [unwired: 11 in]
          n93 = call "BRig_dataLC_Cue2_First_OnOff_l1.vi"() -> ("output_Cue2_First_OnOff"=w187:i32)  [unwired: 11 in]
          n94 = call "BRig_dataLC_Cue2_First_Block_l1.vi"() -> ("output_Cue2_First_Block"=w186:i32)  [unwired: 11 in]
          n95 = call "BRig_dataLC_Cue2_First_Prob_l1.vi"() -> ("output_Cue2_First_Prob"=w185:i32)  [unwired: 11 in]
          n96 = call "BRig_dataLC_Cue2_First_Delay_l1.vi"() -> ("output_Cue2_First_Delay"=w184:i32)  [unwired: 11 in]
          n97 = call "BRig_dataLC_Cue2_First_DelayOpt_l1.vi"() -> ("output_Cue2_First_DelayOpt"=w183:i32)  [unwired: 11 in]
          n98 = call "BRig_dataLC_Cue2_First_Count_l1.vi"() -> ("output_Cue2_First_Count"=w182:i32)  [unwired: 11 in]
          n99 = call "BRig_dataLC_Cue2_PreR_OnOff_l1.vi"() -> ("output_Cue2_PreR_OnOff"=w181:i32)  [unwired: 11 in]
          n100 = call "BRig_dataLC_Cue2_PreR_Block_l1.vi"() -> ("output_Cue2_PreR_Block"=w180:i32)  [unwired: 11 in]
          n101 = call "BRig_dataLC_Cue2_PreR_Prob_l1.vi"() -> ("output_Cue2_PreR_Prob"=w179:i32)  [unwired: 11 in]
          n102 = call "BRig_dataLC_Cue2_PreR_Delay_l1.vi"() -> ("output_Cue2_PreR_Delay"=w178:i32)  [unwired: 11 in]
          n103 = call "BRig_dataLC_Cue2_PreR_DelayOpt_l1.vi"() -> ("output_Cue2_PreR_DelayOpt"=w177:i32)  [unwired: 11 in]
          n104 = call "BRig_dataLC_Cue2_PreR_Count_l1.vi"() -> ("output_Cue2_PreR_Count"=w176:i32)  [unwired: 11 in]
          n105 = call "BRig_dataLC_Cue2_PostR_OnOff_l1.vi"() -> ("output_Cue2_PostR_OnOff"=w175:i32)  [unwired: 11 in]
          n106 = call "BRig_dataLC_Cue2_PostR_Block_l1.vi"() -> ("output_Cue2_PostR_Block"=w174:i32)  [unwired: 11 in]
          n107 = call "BRig_dataLC_Cue2_PostR_Prob_l1.vi"() -> ("output_Cue2_PostR_Prob"=w173:i32)  [unwired: 11 in]
          n108 = call "BRig_dataLC_Cue2_PostR_Delay_l1.vi"() -> ("output_Cue2_PostR_Delay"=w172:i32)  [unwired: 11 in]
          n109 = call "BRig_dataLC_Cue2_PostR_DelayOpt_l1.vi"() -> ("output_Cue2_PostR_DelayOpt"=w171:i32)  [unwired: 11 in]
          n110 = call "BRig_dataLC_Cue2_PostR_Count_l1.vi"() -> ("output_Cue2_PostR_Count"=w170:i32)  [unwired: 11 in]
          n111 = Boolean To (0,1)(Boolean="LC_Cue_First_OnOff") -> (0, 1=w226:i16)
          n112 = Boolean To (0,1)(Boolean="LC_Cue_First_delayOpt") -> (0, 1=w225:i16)
          n113 = Boolean To (0,1)(Boolean="LC_Cue_PreR_OnOff") -> (0, 1=w224:i16)
          n114 = Boolean To (0,1)(Boolean="LC_Cue_PreR_delayOpt") -> (0, 1=w223:i16)
          n115 = Boolean To (0,1)(Boolean="LC_Cue_PostR_OnOff") -> (0, 1=w222:i16)
          n116 = Boolean To (0,1)(Boolean="LC_Cue_PostR_delayOpt") -> (0, 1=w221:i16)
          n117 = Boolean To (0,1)(Boolean="LC_Cue2_First_OnOff") -> (0, 1=w169:i16)
          n118 = Boolean To (0,1)(Boolean="LC_Cue2_First_delayOpt") -> (0, 1=w168:i16)
          n119 = Boolean To (0,1)(Boolean="LC_Cue2_PreR_OnOff") -> (0, 1=w167:i16)
          n120 = Boolean To (0,1)(Boolean="LC_Cue2_PreR_delayOpt") -> (0, 1=w166:i16)
          n121 = Boolean To (0,1)(Boolean="LC_Cue2_PostR_OnOff") -> (0, 1=w165:i16)
          n122 = Boolean To (0,1)(Boolean="LC_Cue2_PostR_delayOpt") -> (0, 1=w164:i16)
          n123 = To Unsigned Word Integer(number=w226) -> (unsigned 16bit integer=w220:u16)
          n124 = To Unsigned Word Integer(number=w225) -> (unsigned 16bit integer=w216:u16)
          n125 = To Unsigned Word Integer(number=w224) -> (unsigned 16bit integer=w214:u16)
          n126 = To Unsigned Word Integer(number=w223) -> (unsigned 16bit integer=w210:u16)
          n127 = To Unsigned Word Integer(number=w222) -> (unsigned 16bit integer=w208:u16)
          n128 = To Unsigned Word Integer(number=w221) -> (unsigned 16bit integer=w204:u16)
          n129 = To Unsigned Word Integer(number=w169) -> (unsigned 16bit integer=w157:u16)
          n130 = To Unsigned Word Integer(number=w168) -> (unsigned 16bit integer=w153:u16)
          n131 = To Unsigned Word Integer(number=w167) -> (unsigned 16bit integer=w151:u16)
          n132 = To Unsigned Word Integer(number=w166) -> (unsigned 16bit integer=w147:u16)
          n133 = To Unsigned Word Integer(number=w165) -> (unsigned 16bit integer=w145:u16)
          n134 = To Unsigned Word Integer(number=w164) -> (unsigned 16bit integer=w141:u16)
          n135 = call "BRig_dataLC_Cue_PostR_nRew1_l1.vi"() -> ("output_Cue_PostR_nRew1_l1"=w139:i32)  [unwired: 11 in]
          n136 = call "BRig_dataLC_Cue_PostR_nRew2_l1.vi"() -> ("output_Cue_PostR_nRew2_l1"=w138:i32)  [unwired: 11 in]
          n137 = call "BRig_dataLC_Cue2_PostR_nRew1_l1.vi"() -> ("output_Cue2_PostR_nRew1_l1"=w137:i32)  [unwired: 11 in]
          n138 = call "BRig_dataLC_Cue2_PostR_nRew2_l1.vi"() -> ("output_Cue2_PostR_nRew2_l1"=w136:i32)  [unwired: 11 in]
          n139 = Replace Array Subset(array=w240, new element #1=w201, index #1=w202, new element #2=w220, index #2=w238, new element #3="LC_Cue_First_Block", index #3=w237, new element #4="LC_Cue_First_Probability", index #4=w236, new element #5="LC_Cue_First_Tdelay", index #5=w235, new element #6=w216, index #6=w234, new element #7="LC_Cue_First_Count", index #7=w233, new element #8=w214, index #8=w198, new element #9="LC_Cue_PreR_Block", index #9=w197, new element #10="LC_Cue_PreR_Probability", index #10=w196, new element #11="LC_Cue_PreR_Tdelay", index #11=w195, new element #12=w210, index #12=w194, new element #13="LC_Cue_PreR_Count", index #13=w199, new element #14=w208, index #14=w200, new element #15="LC_Cue_PostR_Block", index #15=w193, new element #16="LC_Cue_PostR_Probability", index #16=w192, new element #17="LC_Cue_PostR_Tdelay", index #17=w191, new element #18=w204, index #18=w190, new element #19="LC_Cue_PostR_Count", index #19=w189, new element #20=w157, index #20=w187, new element #21="LC_Cue2_First_Block", index #21=w186, new element #22="LC_Cue2_First_Probability", index #22=w185, new element #23="LC_Cue2_First_Tdelay", index #23=w184, new element #24=w153, index #24=w183, new element #25="LC_Cue2_First_Count", index #25=w182, new element #26=w151, index #26=w181, new element #27="LC_Cue2_PreR_Block", index #27=w180, new element #28="LC_Cue2_PreR_Probability", index #28=w179, new element #29="LC_Cue2_PreR_Tdelay", index #29=w178, new element #30=w147, index #30=w177, new element #31="LC_Cue2_PreR_Count", index #31=w176, new element #32=w145, index #32=w175, new element #33="LC_Cue2_PostR_Block", index #33=w174, new element #34="LC_Cue2_PostR_Probability", index #34=w173, new element #35="LC_Cue2_PostR_Tdelay", index #35=w172, new element #36=w141, index #36=w171, new element #37="LC_Cue2_PostR_Count", index #37=w170, new element #38="LC_Cue_nRew1", index #38=w139, new element #39="LC_Cue_nRew2", index #39=w138, new element #40="LC_Cue2_nRew1", index #40=w137, new element #41="LC_Cue2_nRew2", index #41=w136) -> (w239:u16[])
        }
        frame 3 {
          n140 = call "BRig_dataLC_Selection_PostR_OnOff_l1.vi"() -> ("output_Selection_PostR_OnOff"=w257:i32)  [unwired: 11 in]
          n141 = call "BRig_dataLC_Selection_PostR_Block_l1.vi"() -> ("output_Selection_PostR_Block"=w256:i32)  [unwired: 11 in]
          n142 = call "BRig_dataLC_Selection_PostR_Prob_l1.vi"() -> ("output_Selection_PostR_Prob"=w255:i32)  [unwired: 11 in]
          n143 = call "BRig_dataLC_Selection_PostR_Delay_l1.vi"() -> ("output_Selection_PostR_Delay"=w254:i32)  [unwired: 11 in]
          n144 = call "BRig_dataLC_Selection_PostR_Count_l1.vi"() -> ("output_Selection_PostR_Count"=w253:i32)  [unwired: 11 in]
          n145 = call "BRig_dataLC_Selection_PreR_OnOff_l1.vi"() -> ("output_Selection_PreR_OnOff"=w267:i32)  [unwired: 11 in]
          n146 = call "BRig_dataLC_Selection_PreR_Block_l1.vi"() -> ("output_Selection_PreR_Block"=w266:i32)  [unwired: 11 in]
          n147 = call "BRig_dataLC_Selection_PreR_Prob_l1.vi"() -> ("output_Selection_PreR_Prob"=w265:i32)  [unwired: 11 in]
          n148 = call "BRig_dataLC_Selection_PreR_Delay_l1.vi"() -> ("output_Selection_PreR_Delay"=w264:i32)  [unwired: 11 in]
          n149 = call "BRig_dataLC_Selection_PreR_Count_l1.vi"() -> ("output_Selection_PreR_Count"=w263:i32)  [unwired: 11 in]
          n150 = call "BRig_dataLC_Selection_First_OnOff_l1.vi"() -> ("output_Selection_First_OnOff"=w277:i32)  [unwired: 11 in]
          n151 = call "BRig_dataLC_Selection_First_Block_l1.vi"() -> ("output_Selection_First_Block"=w276:i32)  [unwired: 11 in]
          n152 = call "BRig_dataLC_Selection_First_Prob_l1.vi"() -> ("output_Selection_First_Prob"=w275:i32)  [unwired: 11 in]
          n153 = call "BRig_dataLC_Selection_First_Delay_l1.vi"() -> ("output_Selection_First_Delay"=w274:i32)  [unwired: 11 in]
          n154 = call "BRig_dataLC_Selection_First_Count_l1.vi"() -> ("output_Selection_First_Count"=w273:i32)  [unwired: 11 in]
          n155 = Boolean To (0,1)(Boolean="LC_Sel_First_OnOff") -> (0, 1=w280:i16)
          n156 = Boolean To (0,1)(Boolean="LC_Sel_PreR_OnOff") -> (0, 1=w279:i16)
          n157 = Boolean To (0,1)(Boolean="LC_Sel_PostR_OnOff") -> (0, 1=w278:i16)
          n158 = To Unsigned Word Integer(number=w280) -> (unsigned 16bit integer=w272:u16)
          n159 = To Unsigned Word Integer(number=w279) -> (unsigned 16bit integer=w262:u16)
          n160 = To Unsigned Word Integer(number=w278) -> (unsigned 16bit integer=w252:u16)
          n161 = call "BRig_dataLC_Selection_PostR_nRew1_l1.vi"() -> ("output_Selection_PostR_nRew1_l1"=w244:i32)  [unwired: 11 in]
          n162 = call "BRig_dataLC_Selection_PostR_nRew2_l1.vi"() -> ("output_Selection_PostR_nRew2_l1"=w243:i32)  [unwired: 11 in]
          n163 = Replace Array Subset(array=w285, new element #1=w246, index #1=w247, new element #2=w272, index #2=w277, new element #3="LC_Sel_First_Block", index #3=w276, new element #4="LC_Sel_First_Probability", index #4=w275, new element #5="LC_Sel_First_Tdelay", index #5=w274, new element #6="LC_Sel_First_Count", index #6=w273, new element #7=w262, index #7=w267, new element #8="LC_Sel_PreR_Block", index #8=w266, new element #9="LC_Sel_PreR_Probability", index #9=w265, new element #10="LC_Sel_PreR_Tdelay", index #10=w264, new element #11="LC_Sel_PreR_Count", index #11=w263, new element #12=w252, index #12=w257, new element #13="LC_Sel_PostR_Block", index #13=w256, new element #14="LC_Sel_PostR_Probability", index #14=w255, new element #15="LC_Sel_PostR_Tdelay", index #15=w254, new element #16="LC_Sel_PostR_Count", index #16=w253, new element #17="LC_Sel_nRew1", index #17=w244, new element #18="LC_Sel_nRew2", index #18=w243) -> (w284:u16[])
        }
        frame 4 {
          n164 = call "BRig_dataLC_Reward_OnOff_l1.vi"() -> ("output_Reward_OnOff"=w312:i32)  [unwired: 11 in]
          n165 = call "BRig_dataLC_Reward_Block_l1.vi"() -> ("output_Reward_Block"=w311:i32)  [unwired: 11 in]
          n166 = call "BRig_dataLC_Reward_Trial_l1.vi"() -> ("output_Reward_Trial"=w310:i32)  [unwired: 11 in]
          n167 = call "BRig_dataLC_Reward_Prob_l1.vi"() -> ("output_Reward_Prob"=w309:i32)  [unwired: 11 in]
          n168 = call "BRig_dataLC_Reward_Delay_l1.vi"() -> ("output_Reward_Delay"=w308:i32)  [unwired: 11 in]
          n169 = call "BRig_dataLC_Wrong_OnOff_l1.vi"() -> ("output_Wrong_OnOff"=w298:i32)  [unwired: 11 in]
          n170 = call "BRig_dataLC_Wrong_Block_l1.vi"() -> ("output_Wrong_Block"=w297:i32)  [unwired: 11 in]
          n171 = call "BRig_dataLC_Wrong_Trial_l1.vi"() -> ("output_Wrong_Trial"=w296:i32)  [unwired: 11 in]
          n172 = call "BRig_dataLC_Wrong_Prob_l1.vi"() -> ("output_Wrong_Prob"=w295:i32)  [unwired: 11 in]
          n173 = call "BRig_dataLC_Wrong_Delay_l1.vi"() -> ("output_Wrong_Delay"=w294:i32)  [unwired: 11 in]
          n174 = Boolean To (0,1)(Boolean="LC_Reward_OnOff") -> (0, 1=w305:i16)
          n175 = Boolean To (0,1)(Boolean="LC_Wrong_OnOff") -> (0, 1=w304:i16)
          n176 = To Unsigned Word Integer(number=w305) -> (unsigned 16bit integer=w303:u16)
          n177 = To Unsigned Word Integer(number=w304) -> (unsigned 16bit integer=w293:u16)
          n178 = Replace Array Subset(array=w314, new element #1=w287, index #1=w288, new element #2=w303, index #2=w312, new element #3="LC_Reward_Block", index #3=w311, new element #4="LC_Reward_Trial", index #4=w310, new element #5="LC_Reward_Probability", index #5=w309, new element #6="LC_Reward_Tdelay", index #6=w308, new element #7=w293, index #7=w298, new element #8="LC_Wrong_Block", index #8=w297, new element #9="LC_Wrong_Trial", index #9=w296, new element #10="LC_Wrong_Probability", index #10=w295, new element #11="LC_Wrong_Tdelay", index #11=w294) -> (w313:u16[])
        }
        frame 5 {
          w338 = 100.0 ("y")
          n179 = call "BRig_dataExp_LED_baseline_l1.vi"() -> ("output_LED_baseline_l1"=w315:i32)  [unwired: 11 in]
          n180 = call "BRig_dataExp_L_freq_l1.vi"() -> ("output_L_freq_l1"=w337:i32)  [unwired: 11 in]
          n181 = call "BRig_dataExp_L_T_l1.vi"() -> ("output_L_T_l1"=w336:i32)  [unwired: 11 in]
          n182 = call "BRig_dataExp_L_Tpeak_l1.vi"() -> ("output_L_Tpeak_l1"=w335:i32)  [unwired: 11 in]
          n183 = call "BRig_dataExp_L_Tshutter_l1.vi"() -> ("output_L_Tshutter_l1"=w334:i32)  [unwired: 11 in]
          n184 = call "BRig_dataExp_L_power_min_l1.vi"() -> ("output_L_power_min_l1"=w333:i32)  [unwired: 11 in]
          n185 = call "BRig_dataExp_L_power_max_l1.vi"() -> ("output_L_power_max_l1"=w332:i32)  [unwired: 11 in]
          n186 = call "BRig_dataExp_L_power_step_l1.vi"() -> ("output_L_power_step_l1"=w331:i32)  [unwired: 11 in]
          n187 = call "BRig_dataExp_L_Ttotal_l1.vi"() -> ("output_L_Ttotal_l1"=w325:i32)  [unwired: 11 in]
          n188 = Boolean To (0,1)(Boolean="LED_baseline") -> (0, 1=w350:i16)
          n189 = To Unsigned Word Integer(number=w350) -> (unsigned 16bit integer=w348:u16)
          n190 = Multiply(x="Laser_power_min", y=w338) -> (x*y=w342:dbl)
          n191 = Multiply(x="Laser_power_max", y=w338) -> (x*y=w344:dbl)
          n192 = Multiply(x="Laser_power_step", y=w338) -> (x*y=w347:dbl)
          n193 = Round To Nearest(number=w342) -> (nearest integer value=w341:dbl)
          n194 = Round To Nearest(number=w344) -> (nearest integer value=w343:dbl)
          n195 = Round To Nearest(number=w347) -> (nearest integer value=w346:dbl)
          n196 = To Unsigned Word Integer(number=w341) -> (unsigned 16bit integer=w328:u16)
          n197 = To Unsigned Word Integer(number=w343) -> (unsigned 16bit integer=w329:u16)
          n198 = To Unsigned Word Integer(number=w346) -> (unsigned 16bit integer=w330:u16)
          n199 = Add(x="Laser_T", y="Laser_Tshutter") -> (x+y=w322:u16)
          n200 = Replace Array Subset(array=w319, new element=w316, index=w317) -> (w318:u16[])
          n201 = Replace Array Subset(array=w321, new element #1=w348, index #1=w315, new element #2="Laser_Freq", index #2=w337, new element #3="Laser_T", index #3=w336, new element #4="Laser_Tpeak", index #4=w335, new element #5="Laser_Tshutter", index #5=w334, new element #6=w328, index #6=w333, new element #7=w329, index #7=w332, new element #8=w330, index #8=w331, new element #9=w322, index #9=w325) -> (w320:u16[])
        }
        frame 6 {
          n202 = call "BRig_dataExp_L_freq_l1.vi"() -> ("output_L_freq_l1"=w353:i32)  [unwired: 11 in]
          n203 = call "BRig_dataExp_L_T_l1.vi"() -> ("output_L_T_l1"=w354:i32)  [unwired: 11 in]
          n204 = call "BRig_dataExp_L_Tpeak_l1.vi"() -> ("output_L_Tpeak_l1"=w352:i32)  [unwired: 11 in]
          n205 = call "BRig_dataExp_L_Tshutter_l1.vi"() -> ("output_L_Tshutter_l1"=w351:i32)  [unwired: 11 in]
          n206 = Replace Array Subset(array=w358, new element=w355, index=w356) -> (w357:u16[])
          n207 = call "BRig_RT__Case_Idle__calc_LaserPulse.vi"("input_dataExp_L_Tshutter"=w351, "input_dataExp_L_Tpeak"=w352, "input_dataExp_L_T"=w354, "input_dataExp_L_freq"=w353, "input_dataExp"=w360) -> ("output_cluster"=→"LaserPulseTrain":cluster{u16[], u16[]})  [unwired: 6 in]
        }
      }
    }
    frame True {
      w481 = 100.0 ("y")
      n208 = call "BRig_dataLC_ENL_First_OnOff_l1.vi"() -> ("output_ENL_First_OnOff"=w623:i32)  [unwired: 11 in]
      n209 = call "BRig_dataLC_ENL_First_Block_l1.vi"() -> ("output_ENL_First_Block"=w622:i32)  [unwired: 11 in]
      n210 = call "BRig_dataLC_ENL_First_Prob_l1.vi"() -> ("output_ENL_First_Prob"=w621:i32)  [unwired: 11 in]
      n211 = call "BRig_dataLC_ENL_First_Delay_l1.vi"() -> ("output_ENL_First_Delay"=w620:i32)  [unwired: 11 in]
      n212 = call "BRig_dataLC_ENL_First_DelayOpt_l1.vi"() -> ("output_ENL_First_DelayOpt"=w619:i32)  [unwired: 11 in]
      n213 = call "BRig_dataLC_ENL_First_Count_l1.vi"() -> ("output_ENL_First_Count"=w618:i32)  [unwired: 11 in]
      n214 = call "BRig_dataLC_ENL_PreR_OnOff_l1.vi"() -> ("output_ENL_PreR_OnOff"=w617:i32)  [unwired: 11 in]
      n215 = call "BRig_dataLC_ENL_PreR_Block_l1.vi"() -> ("output_ENL_PreR_Block"=w616:i32)  [unwired: 11 in]
      n216 = call "BRig_dataLC_ENL_PreR_Prob_l1.vi"() -> ("output_ENL_PreR_Prob"=w615:i32)  [unwired: 11 in]
      n217 = call "BRig_dataLC_ENL_PreR_Delay_l1.vi"() -> ("output_ENL_PreR_Delay"=w614:i32)  [unwired: 11 in]
      n218 = call "BRig_dataLC_ENL_PreR_DelayOpt_l1.vi"() -> ("output_ENL_PreR_DelayOpt"=w613:i32)  [unwired: 11 in]
      n219 = call "BRig_dataLC_ENL_PreR_Count_l1.vi"() -> ("output_ENL_PreR_Count"=w612:i32)  [unwired: 11 in]
      n220 = call "BRig_dataLC_ENL_PostR_OnOff_l1.vi"() -> ("output_ENL_PostR_OnOff"=w611:i32)  [unwired: 11 in]
      n221 = call "BRig_dataLC_ENL_PostR_Block_l1.vi"() -> ("output_ENL_PostR_Block"=w610:i32)  [unwired: 11 in]
      n222 = call "BRig_dataLC_ENL_PostR_Prob_l1.vi"() -> ("output_ENL_PostR_Prob"=w609:i32)  [unwired: 11 in]
      n223 = call "BRig_dataLC_ENL_PostR_Delay_l1.vi"() -> ("output_ENL_PostR_Delay"=w608:i32)  [unwired: 11 in]
      n224 = call "BRig_dataLC_ENL_PostR_DelayOpt_l1.vi"() -> ("output_ENL_PostR_DelayOpt"=w607:i32)  [unwired: 11 in]
      n225 = call "BRig_dataLC_ENL_PostR_Count_l1.vi"() -> ("output_ENL_PostR_Count"=w606:i32)  [unwired: 11 in]
      n226 = call "BRig_dataLC_ENL2_First_OnOff_l1.vi"() -> ("output_ENL2_First_OnOff"=w466:i32)  [unwired: 11 in]
      n227 = call "BRig_dataLC_ENL2_First_Block_l1.vi"() -> ("output_ENL2_First_Block"=w465:i32)  [unwired: 11 in]
      n228 = call "BRig_dataLC_ENL2_First_Prob_l1.vi"() -> ("output_ENL2_First_Prob"=w464:i32)  [unwired: 11 in]
      n229 = call "BRig_dataLC_ENL2_First_Delay_l1.vi"() -> ("output_ENL2_First_Delay"=w463:i32)  [unwired: 11 in]
      n230 = call "BRig_dataLC_ENL2_First_DelayOpt_l1.vi"() -> ("output_ENL2_First_DelayOpt"=w462:i32)  [unwired: 11 in]
      n231 = call "BRig_dataLC_ENL2_First_Count_l1.vi"() -> ("output_ENL2_First_Count"=w461:i32)  [unwired: 11 in]
      n232 = call "BRig_dataLC_ENL2_PreR_OnOff_l1.vi"() -> ("output_ENL2_PreR_OnOff"=w460:i32)  [unwired: 11 in]
      n233 = call "BRig_dataLC_ENL2_PreR_Block_l1.vi"() -> ("output_ENL2_PreR_Block"=w459:i32)  [unwired: 11 in]
      n234 = call "BRig_dataLC_ENL2_PreR_Prob_l1.vi"() -> ("output_ENL2_PreR_Prob"=w458:i32)  [unwired: 11 in]
      n235 = call "BRig_dataLC_ENL2_PreR_Delay_l1.vi"() -> ("output_ENL2_PreR_Delay"=w457:i32)  [unwired: 11 in]
      n236 = call "BRig_dataLC_ENL2_PreR_DelayOpt_l1.vi"() -> ("output_ENL2_PreR_DelayOpt"=w456:i32)  [unwired: 11 in]
      n237 = call "BRig_dataLC_ENL2_PreR_Count_l1.vi"() -> ("output_ENL2_PreR_Count"=w455:i32)  [unwired: 11 in]
      n238 = call "BRig_dataLC_ENL2_PostR_OnOff_l1.vi"() -> ("output_ENL2_PostR_OnOff"=w454:i32)  [unwired: 11 in]
      n239 = call "BRig_dataLC_ENL2_PostR_Block_l1.vi"() -> ("output_ENL2_PostR_Block"=w453:i32)  [unwired: 11 in]
      n240 = call "BRig_dataLC_ENL2_PostR_Prob_l1.vi"() -> ("output_ENL2_PostR_Prob"=w452:i32)  [unwired: 11 in]
      n241 = call "BRig_dataLC_ENL2_PostR_Delay_l1.vi"() -> ("output_ENL2_PostR_Delay"=w451:i32)  [unwired: 11 in]
      n242 = call "BRig_dataLC_ENL2_PostR_DelayOpt_l1.vi"() -> ("output_ENL2_PostR_DelayOpt"=w450:i32)  [unwired: 11 in]
      n243 = call "BRig_dataLC_ENL2_PostR_Count_l1.vi"() -> ("output_ENL2_PostR_Count"=w449:i32)  [unwired: 11 in]
      n244 = Index Array(array=w378, index #1=w623, index #2=w622, index #3=w621, index #4=w620, index #5=w619, index #6=w618, index #7=w617, index #8=w616, index #9=w615, index #10=w614, index #11=w613, index #12=w612, index #13=w611, index #14=w610, index #15=w609, index #16=w608, index #17=w607, index #18=w606) -> (element #1=w599:u16, element #2=w598:u16, element #3=w597:u16, element #4=w596:u16, element #5=w595:u16, element #6=w594:u16, element #7=w593:u16, element #8=w592:u16, element #9=w591:u16, element #10=w590:u16, element #11=w589:u16, element #12=w588:u16, element #13=w587:u16, element #14=w586:u16, element #15=w585:u16, element #16=w584:u16, element #17=w583:u16, element #18=w582:u16)
      n245 = Index Array(array=w378, index #1=w466, index #2=w465, index #3=w464, index #4=w463, index #5=w462, index #6=w461, index #7=w460, index #8=w459, index #9=w458, index #10=w457, index #11=w456, index #12=w455, index #13=w454, index #14=w453, index #15=w452, index #16=w451, index #17=w450, index #18=w449) -> (element #1=w425:u16, element #2=w426:u16, element #3=w427:u16, element #4=w428:u16, element #5=w429:u16, element #6=w430:u16, element #7=w431:u16, element #8=w432:u16, element #9=w433:u16, element #10=w434:u16, element #11=w435:u16, element #12=w436:u16, element #13=w438:u16, element #14=w439:u16, element #15=w440:u16, element #16=w441:u16, element #17=w442:u16, element #18=w443:u16)
      n246 = Not Equal To 0?(x=w599) -> (x != 0?=w605:bool)
      n247 = Not Equal To 0?(x=w595) -> (x != 0?=w604:bool)
      n248 = Not Equal To 0?(x=w593) -> (x != 0?=w603:bool)
      n249 = Not Equal To 0?(x=w589) -> (x != 0?=w602:bool)
      n250 = Not Equal To 0?(x=w587) -> (x != 0?=w601:bool)
      n251 = Not Equal To 0?(x=w583) -> (x != 0?=w600:bool)
      n252 = local write "LC_ENL_First_OnOff"(w605) -> ()
      n253 = local write "LC_ENL_First_Block"(w598) -> ()
      n254 = local write "LC_ENL_First_Probability"(w597) -> ()
      n255 = local write "LC_ENL_First_Tdelay"(w596) -> ()
      n256 = local write "LC_ENL_First_delayOpt"(w604) -> ()
      n257 = local write "LC_ENL_First_Count"(w594) -> ()
      n258 = local write "LC_ENL_PreR_OnOff"(w603) -> ()
      n259 = local write "LC_ENL_PreR_Block"(w592) -> ()
      n260 = local write "LC_ENL_PreR_Probability"(w591) -> ()
      n261 = local write "LC_ENL_PreR_Tdelay"(w590) -> ()
      n262 = local write "LC_ENL_PreR_delayOpt"(w602) -> ()
      n263 = local write "LC_ENL_PreR_Count"(w588) -> ()
      n264 = local write "LC_ENL_PostR_OnOff"(w601) -> ()
      n265 = local write "LC_ENL_PostR_Block"(w586) -> ()
      n266 = local write "LC_ENL_PostR_Probability"(w585) -> ()
      n267 = local write "LC_ENL_PostR_Tdelay"(w584) -> ()
      n268 = local write "LC_ENL_PostR_delayOpt"(w600) -> ()
      n269 = local write "LC_ENL_PostR_Count"(w582) -> ()
      n270 = Not Equal To 0?(x=w425) -> (x != 0?=w446:bool)
      n271 = Not Equal To 0?(x=w429) -> (x != 0?=w447:bool)
      n272 = Not Equal To 0?(x=w431) -> (x != 0?=w445:bool)
      n273 = Not Equal To 0?(x=w435) -> (x != 0?=w448:bool)
      n274 = Not Equal To 0?(x=w438) -> (x != 0?=w444:bool)
      n275 = Not Equal To 0?(x=w442) -> (x != 0?=w437:bool)
      n276 = local write "LC_ENL2_First_OnOff"(w446) -> ()
      n277 = local write "LC_ENL2_First_Block"(w426) -> ()
      n278 = local write "LC_ENL2_First_Probability"(w427) -> ()
      n279 = local write "LC_ENL2_First_Tdelay"(w428) -> ()
      n280 = local write "LC_ENL2_First_delayOpt"(w447) -> ()
      n281 = local write "LC_ENL2_First_Count"(w430) -> ()
      n282 = local write "LC_ENL2_PreR_OnOff"(w445) -> ()
      n283 = local write "LC_ENL2_PreR_Block"(w432) -> ()
      n284 = local write "LC_ENL2_PreR_Probability"(w433) -> ()
      n285 = local write "LC_ENL2_PreR_Tdelay"(w434) -> ()
      n286 = local write "LC_ENL2_PreR_delayOpt"(w448) -> ()
      n287 = local write "LC_ENL2_PreR_Count"(w436) -> ()
      n288 = local write "LC_ENL2_PostR_OnOff"(w444) -> ()
      n289 = local write "LC_ENL2_PostR_Block"(w439) -> ()
      n290 = local write "LC_ENL2_PostR_Probability"(w440) -> ()
      n291 = local write "LC_ENL2_PostR_Tdelay"(w441) -> ()
      n292 = local write "LC_ENL2_PostR_delayOpt"(w437) -> ()
      n293 = local write "LC_ENL2_PostR_Count"(w443) -> ()
      n294 = call "BRig_dataLC_Cue_PreR_OnOff_l1.vi"() -> ("output_Cue_PreR_OnOff"=w471:i32)  [unwired: 11 in]
      n295 = call "BRig_dataLC_Cue_PreR_Block_l1.vi"() -> ("output_Cue_PreR_Block"=w470:i32)  [unwired: 11 in]
      n296 = call "BRig_dataLC_Cue_PreR_Prob_l1.vi"() -> ("output_Cue_PreR_Prob"=w469:i32)  [unwired: 11 in]
      n297 = call "BRig_dataLC_Cue_PreR_Delay_l1.vi"() -> ("output_Cue_PreR_Delay"=w468:i32)  [unwired: 11 in]
      n298 = call "BRig_dataLC_Cue_PreR_DelayOpt_l1.vi"() -> ("output_Cue_PreR_DelayOpt"=w467:i32)  [unwired: 11 in]
      n299 = call "BRig_dataLC_Cue_PreR_Count_l1.vi"() -> ("output_Cue_PreR_Count"=w472:i32)  [unwired: 11 in]
      n300 = call "BRig_dataLC_Cue_First_OnOff_l1.vi"() -> ("output_Cue_First_OnOff"=w629:i32)  [unwired: 11 in]
      n301 = call "BRig_dataLC_Cue_First_Block_l1.vi"() -> ("output_Cue_First_Block"=w628:i32)  [unwired: 11 in]
      n302 = call "BRig_dataLC_Cue_First_Prob_l1.vi"() -> ("output_Cue_First_Prob"=w627:i32)  [unwired: 11 in]
      n303 = call "BRig_dataLC_Cue_First_Delay_l1.vi"() -> ("output_Cue_First_Delay"=w626:i32)  [unwired: 11 in]
      n304 = call "BRig_dataLC_Cue_First_DelayOpt_l1.vi"() -> ("output_Cue_First_DelayOpt"=w625:i32)  [unwired: 11 in]
      n305 = call "BRig_dataLC_Cue_First_Count_l1.vi"() -> ("output_Cue_First_Count"=w624:i32)  [unwired: 11 in]
      n306 = call "BRig_dataLC_Cue_PostR_OnOff_l1.vi"() -> ("output_Cue_PostR_OnOff"=w477:i32)  [unwired: 11 in]
      n307 = call "BRig_dataLC_Cue_PostR_Block_l1.vi"() -> ("output_Cue_PostR_Block"=w476:i32)  [unwired: 11 in]
      n308 = call "BRig_dataLC_Cue_PostR_Prob_l1.vi"() -> ("output_Cue_PostR_Prob"=w475:i32)  [unwired: 11 in]
      n309 = call "BRig_dataLC_Cue_PostR_Delay_l1.vi"() -> ("output_Cue_PostR_Delay"=w474:i32)  [unwired: 11 in]
      n310 = call "BRig_dataLC_Cue_PostR_DelayOpt_l1.vi"() -> ("output_Cue_PostR_DelayOpt"=w473:i32)  [unwired: 11 in]
      n311 = call "BRig_dataLC_Cue_PostR_Count_l1.vi"() -> ("output_Cue_PostR_Count"=w478:i32)  [unwired: 11 in]
      n312 = call "BRig_dataExp_LED_baseline_Cue.vi"() -> ("output_LED_baseline_Cue"=w502:i32)  [unwired: 11 in]
      n313 = call "BRig_dataExp_L_freq_l1.vi"() -> ("output_L_freq_l1"=w501:i32)  [unwired: 11 in]
      n314 = call "BRig_dataExp_L_T_l1.vi"() -> ("output_L_T_l1"=w500:i32)  [unwired: 11 in]
      n315 = call "BRig_dataExp_L_Tpeak_l1.vi"() -> ("output_L_Tpeak_l1"=w499:i32)  [unwired: 11 in]
      n316 = call "BRig_dataExp_L_Tshutter_l1.vi"() -> ("output_L_Tshutter_l1"=w498:i32)  [unwired: 11 in]
      n317 = call "BRig_dataExp_L_power_min_l1.vi"() -> ("output_L_power_min_l1"=w497:i32)  [unwired: 11 in]
      n318 = call "BRig_dataExp_L_power_max_l1.vi"() -> ("output_L_power_max_l1"=w496:i32)  [unwired: 11 in]
      n319 = call "BRig_dataExp_L_power_step_l1.vi"() -> ("output_L_power_step_l1"=w495:i32)  [unwired: 11 in]
      n320 = Index Array(array=w378, index #1=w629, index #2=w628, index #3=w627, index #4=w626, index #5=w625, index #6=w624, index #7=w471, index #8=w470, index #9=w469, index #10=w468, index #11=w467, index #12=w472, index #13=w477, index #14=w476, index #15=w475, index #16=w474, index #17=w473, index #18=w478) -> (element #1=w575:u16, element #2=w574:u16, element #3=w573:u16, element #4=w572:u16, element #5=w571:u16, element #6=w570:u16, element #7=w569:u16, element #8=w568:u16, element #9=w567:u16, element #10=w566:u16, element #11=w565:u16, element #12=w564:u16, element #13=w563:u16, element #14=w562:u16, element #15=w561:u16, element #16=w560:u16, element #17=w559:u16, element #18=w558:u16)
      n321 = Index Array(array=w377, index #1=w502, index #2=w501, index #3=w500, index #4=w499, index #5=w498, index #6=w497, index #7=w496, index #8=w495) -> (element #1=w494:u16, element #2=w492:u16, element #3=w491:u16, element #4=w490:u16, element #5=w489:u16, element #6=w488:u16, element #7=w487:u16, element #8=w486:u16)
      n322 = To Double Precision Float(number=w488) -> (double precision float=w485:dbl)
      n323 = To Double Precision Float(number=w487) -> (double precision float=w480:dbl)
      n324 = To Double Precision Float(number=w486) -> (double precision float=w479:dbl)
      n325 = Not Equal To 0?(x=w575) -> (x != 0?=w581:bool)
      n326 = Not Equal To 0?(x=w571) -> (x != 0?=w580:bool)
      n327 = Not Equal To 0?(x=w569) -> (x != 0?=w579:bool)
      n328 = Not Equal To 0?(x=w565) -> (x != 0?=w578:bool)
      n329 = Not Equal To 0?(x=w563) -> (x != 0?=w577:bool)
      n330 = Not Equal To 0?(x=w559) -> (x != 0?=w576:bool)
      n331 = Divide(x=w485, y=w481) -> (x/y=w484:dbl)
      n332 = Divide(x=w480, y=w481) -> (x/y=w483:dbl)
      n333 = Divide(x=w479, y=w481) -> (x/y=w482:dbl)
      n334 = local write "LC_Cue_First_OnOff"(w581) -> ()
      n335 = local write "LC_Cue_First_Block"(w574) -> ()
      n336 = local write "LC_Cue_First_Probability"(w573) -> ()
      n337 = local write "LC_Cue_First_Tdelay"(w572) -> ()
      n338 = local write "LC_Cue_First_delayOpt"(w580) -> ()
      n339 = local write "LC_Cue_First_Count"(w570) -> ()
      n340 = local write "LC_Cue_PreR_OnOff"(w579) -> ()
      n341 = local write "LC_Cue_PreR_Block"(w568) -> ()
      n342 = local write "LC_Cue_PreR_Probability"(w567) -> ()
      n343 = local write "LC_Cue_PreR_Tdelay"(w566) -> ()
      n344 = local write "LC_Cue_PreR_delayOpt"(w578) -> ()
      n345 = local write "LC_Cue_PreR_Count"(w564) -> ()
      n346 = local write "LC_Cue_PostR_OnOff"(w577) -> ()
      n347 = local write "LC_Cue_PostR_Block"(w562) -> ()
      n348 = local write "LC_Cue_PostR_Probability"(w561) -> ()
      n349 = local write "LC_Cue_PostR_Tdelay"(w560) -> ()
      n350 = local write "LC_Cue_PostR_delayOpt"(w576) -> ()
      n351 = local write "LC_Cue_PostR_Count"(w558) -> ()
      n352 = Not Equal To 0?(x=w494) -> (x != 0?=w493:bool)
      n353 = call "BRig_dataLC_Cue2_First_OnOff_l1.vi"() -> ("output_Cue2_First_OnOff"=w401:i32)  [unwired: 11 in]
      n354 = call "BRig_dataLC_Cue2_First_Block_l1.vi"() -> ("output_Cue2_First_Block"=w402:i32)  [unwired: 11 in]
      n355 = call "BRig_dataLC_Cue2_First_Prob_l1.vi"() -> ("output_Cue2_First_Prob"=w403:i32)  [unwired: 11 in]
      n356 = call "BRig_dataLC_Cue2_First_Delay_l1.vi"() -> ("output_Cue2_First_Delay"=w404:i32)  [unwired: 11 in]
      n357 = call "BRig_dataLC_Cue2_First_DelayOpt_l1.vi"() -> ("output_Cue2_First_DelayOpt"=w405:i32)  [unwired: 11 in]
      n358 = call "BRig_dataLC_Cue2_First_Count_l1.vi"() -> ("output_Cue2_First_Count"=w406:i32)  [unwired: 11 in]
      n359 = call "BRig_dataLC_Cue2_PreR_OnOff_l1.vi"() -> ("output_Cue2_PreR_OnOff"=w407:i32)  [unwired: 11 in]
      n360 = call "BRig_dataLC_Cue2_PreR_Block_l1.vi"() -> ("output_Cue2_PreR_Block"=w408:i32)  [unwired: 11 in]
      n361 = call "BRig_dataLC_Cue2_PreR_Prob_l1.vi"() -> ("output_Cue2_PreR_Prob"=w409:i32)  [unwired: 11 in]
      n362 = call "BRig_dataLC_Cue2_PreR_Delay_l1.vi"() -> ("output_Cue2_PreR_Delay"=w410:i32)  [unwired: 11 in]
      n363 = call "BRig_dataLC_Cue2_PreR_DelayOpt_l1.vi"() -> ("output_Cue2_PreR_DelayOpt"=w411:i32)  [unwired: 11 in]
      n364 = call "BRig_dataLC_Cue2_PreR_Count_l1.vi"() -> ("output_Cue2_PreR_Count"=w412:i32)  [unwired: 11 in]
      n365 = call "BRig_dataLC_Cue2_PostR_OnOff_l1.vi"() -> ("output_Cue2_PostR_OnOff"=w413:i32)  [unwired: 11 in]
      n366 = call "BRig_dataLC_Cue2_PostR_Block_l1.vi"() -> ("output_Cue2_PostR_Block"=w414:i32)  [unwired: 11 in]
      n367 = call "BRig_dataLC_Cue2_PostR_Prob_l1.vi"() -> ("output_Cue2_PostR_Prob"=w415:i32)  [unwired: 11 in]
      n368 = call "BRig_dataLC_Cue2_PostR_Delay_l1.vi"() -> ("output_Cue2_PostR_Delay"=w416:i32)  [unwired: 11 in]
      n369 = call "BRig_dataLC_Cue2_PostR_DelayOpt_l1.vi"() -> ("output_Cue2_PostR_DelayOpt"=w417:i32)  [unwired: 11 in]
      n370 = call "BRig_dataLC_Cue2_PostR_Count_l1.vi"() -> ("output_Cue2_PostR_Count"=w418:i32)  [unwired: 11 in]
      n371 = local write "LED_baseline"(w493) -> ()
      n372 = local write "Laser_Freq"(w492) -> ()
      n373 = local write "Laser_T"(w491) -> ()
      n374 = local write "Laser_Tpeak"(w490) -> ()
      n375 = local write "Laser_Tshutter"(w489) -> ()
      n376 = local write "Laser_power_min"(w484) -> ()
      n377 = local write "Laser_power_max"(w483) -> ()
      n378 = local write "Laser_power_step"(w482) -> ()
      n379 = Index Array(array=w378, index #1=w401, index #2=w402, index #3=w403, index #4=w404, index #5=w405, index #6=w406, index #7=w407, index #8=w408, index #9=w409, index #10=w410, index #11=w411, index #12=w412, index #13=w413, index #14=w414, index #15=w415, index #16=w416, index #17=w417, index #18=w418) -> (element #1=w419:u16, element #2=w397:u16, element #3=w396:u16, element #4=w395:u16, element #5=w420:u16, element #6=w398:u16, element #7=w421:u16, element #8=w392:u16, element #9=w391:u16, element #10=w390:u16, element #11=w422:u16, element #12=w389:u16, element #13=w423:u16, element #14=w386:u16, element #15=w385:u16, element #16=w384:u16, element #17=w424:u16, element #18=w383:u16)
      n380 = call "BRig_dataLC_Selection_PostR_OnOff_l1.vi"() -> ("output_Selection_PostR_OnOff"=w547:i32)  [unwired: 11 in]
      n381 = call "BRig_dataLC_Selection_PostR_Block_l1.vi"() -> ("output_Selection_PostR_Block"=w546:i32)  [unwired: 11 in]
      n382 = call "BRig_dataLC_Selection_PostR_Prob_l1.vi"() -> ("output_Selection_PostR_Prob"=w545:i32)  [unwired: 11 in]
      n383 = call "BRig_dataLC_Selection_PostR_Delay_l1.vi"() -> ("output_Selection_PostR_Delay"=w544:i32)  [unwired: 11 in]
      n384 = call "BRig_dataLC_Selection_PostR_Count_l1.vi"() -> ("output_Selection_PostR_Count"=w543:i32)  [unwired: 11 in]
      n385 = call "BRig_dataLC_Selection_PreR_OnOff_l1.vi"() -> ("output_Selection_PreR_OnOff"=w552:i32)  [unwired: 11 in]
      n386 = call "BRig_dataLC_Selection_PreR_Block_l1.vi"() -> ("output_Selection_PreR_Block"=w551:i32)  [unwired: 11 in]
      n387 = call "BRig_dataLC_Selection_PreR_Prob_l1.vi"() -> ("output_Selection_PreR_Prob"=w550:i32)  [unwired: 11 in]
      n388 = call "BRig_dataLC_Selection_PreR_Delay_l1.vi"() -> ("output_Selection_PreR_Delay"=w549:i32)  [unwired: 11 in]
      n389 = call "BRig_dataLC_Selection_PreR_Count_l1.vi"() -> ("output_Selection_PreR_Count"=w548:i32)  [unwired: 11 in]
      n390 = call "BRig_dataLC_Selection_First_OnOff_l1.vi"() -> ("output_Selection_First_OnOff"=w557:i32)  [unwired: 11 in]
      n391 = call "BRig_dataLC_Selection_First_Block_l1.vi"() -> ("output_Selection_First_Block"=w556:i32)  [unwired: 11 in]
      n392 = call "BRig_dataLC_Selection_First_Prob_l1.vi"() -> ("output_Selection_First_Prob"=w555:i32)  [unwired: 11 in]
      n393 = call "BRig_dataLC_Selection_First_Delay_l1.vi"() -> ("output_Selection_First_Delay"=w554:i32)  [unwired: 11 in]
      n394 = call "BRig_dataLC_Selection_First_Count_l1.vi"() -> ("output_Selection_First_Count"=w553:i32)  [unwired: 11 in]
      n395 = call "BRig_dataLC_Reward_OnOff_l1.vi"() -> ("output_Reward_OnOff"=w524:i32)  [unwired: 11 in]
      n396 = call "BRig_dataLC_Reward_Block_l1.vi"() -> ("output_Reward_Block"=w523:i32)  [unwired: 11 in]
      n397 = call "BRig_dataLC_Reward_Trial_l1.vi"() -> ("output_Reward_Trial"=w522:i32)  [unwired: 11 in]
      n398 = call "BRig_dataLC_Reward_Prob_l1.vi"() -> ("output_Reward_Prob"=w521:i32)  [unwired: 11 in]
      n399 = call "BRig_dataLC_Reward_Delay_l1.vi"() -> ("output_Reward_Delay"=w520:i32)  [unwired: 11 in]
      n400 = call "BRig_dataLC_Wrong_OnOff_l1.vi"() -> ("output_Wrong_OnOff"=w519:i32)  [unwired: 11 in]
      n401 = call "BRig_dataLC_Wrong_Block_l1.vi"() -> ("output_Wrong_Block"=w518:i32)  [unwired: 11 in]
      n402 = call "BRig_dataLC_Wrong_Trial_l1.vi"() -> ("output_Wrong_Trial"=w517:i32)  [unwired: 11 in]
      n403 = call "BRig_dataLC_Wrong_Prob_l1.vi"() -> ("output_Wrong_Prob"=w516:i32)  [unwired: 11 in]
      n404 = call "BRig_dataLC_Wrong_Delay_l1.vi"() -> ("output_Wrong_Delay"=w515:i32)  [unwired: 11 in]
      n405 = Not Equal To 0?(x=w419) -> (x != 0?=w400:bool)
      n406 = Not Equal To 0?(x=w420) -> (x != 0?=w399:bool)
      n407 = Not Equal To 0?(x=w421) -> (x != 0?=w393:bool)
      n408 = Not Equal To 0?(x=w422) -> (x != 0?=w394:bool)
      n409 = Not Equal To 0?(x=w423) -> (x != 0?=w388:bool)
      n410 = Not Equal To 0?(x=w424) -> (x != 0?=w387:bool)
      n411 = call "BRig_dataLC_ENL_PostR_nRew1_l1.vi"() -> ("output_ENL_PostR_nRew1_l1"=w382:i32)  [unwired: 11 in]
      n412 = call "BRig_dataLC_ENL_PostR_nRew2_l1.vi"() -> ("output_ENL_PostR_nRew2_l1"=w381:i32)  [unwired: 11 in]
      n413 = call "BRig_dataLC_ENL2_PostR_nRew1_l1.vi"() -> ("output_ENL2_PostR_nRew1_l1"=w376:i32)  [unwired: 11 in]
      n414 = call "BRig_dataLC_ENL2_PostR_nRew2_l1.vi"() -> ("output_ENL2_PostR_nRew2_l1"=w375:i32)  [unwired: 11 in]
      n415 = call "BRig_dataLC_Cue_PostR_nRew1_l1.vi"() -> ("output_Cue_PostR_nRew1_l1"=w372:i32)  [unwired: 11 in]
      n416 = call "BRig_dataLC_Cue_PostR_nRew2_l1.vi"() -> ("output_Cue_PostR_nRew2_l1"=w371:i32)  [unwired: 11 in]
      n417 = call "BRig_dataLC_Cue2_PostR_nRew1_l1.vi"() -> ("output_Cue2_PostR_nRew1_l1"=w370:i32)  [unwired: 11 in]
      n418 = call "BRig_dataLC_Cue2_PostR_nRew2_l1.vi"() -> ("output_Cue2_PostR_nRew2_l1"=w369:i32)  [unwired: 11 in]
      n419 = call "BRig_dataLC_Selection_PostR_nRew1_l1.vi"() -> ("output_Selection_PostR_nRew1_l1"=w368:i32)  [unwired: 11 in]
      n420 = call "BRig_dataLC_Selection_PostR_nRew2_l1.vi"() -> ("output_Selection_PostR_nRew2_l1"=w367:i32)  [unwired: 11 in]
      n421 = Index Array(array=w378, index #1=w524, index #2=w523, index #3=w522, index #4=w521, index #5=w520, index #6=w519, index #7=w518, index #8=w517, index #9=w516, index #10=w515) -> (element #1=w512:u16, element #2=w511:u16, element #3=w510:u16, element #4=w509:u16, element #5=w508:u16, element #6=w507:u16, element #7=w506:u16, element #8=w505:u16, element #9=w504:u16, element #10=w503:u16)
      n422 = local write "LC_Cue2_First_OnOff"(w400) -> ()
      n423 = local write "LC_Cue2_First_Block"(w397) -> ()
      n424 = local write "LC_Cue2_First_Probability"(w396) -> ()
      n425 = local write "LC_Cue2_First_Tdelay"(w395) -> ()
      n426 = local write "LC_Cue2_First_delayOpt"(w399) -> ()
      n427 = local write "LC_Cue2_First_Count"(w398) -> ()
      n428 = local write "LC_Cue2_PreR_OnOff"(w393) -> ()
      n429 = local write "LC_Cue2_PreR_Block"(w392) -> ()
      n430 = local write "LC_Cue2_PreR_Probability"(w391) -> ()
      n431 = local write "LC_Cue2_PreR_Tdelay"(w390) -> ()
      n432 = local write "LC_Cue2_PreR_delayOpt"(w394) -> ()
      n433 = local write "LC_Cue2_PreR_Count"(w389) -> ()
      n434 = local write "LC_Cue2_PostR_OnOff"(w388) -> ()
      n435 = local write "LC_Cue2_PostR_Block"(w386) -> ()
      n436 = local write "LC_Cue2_PostR_Probability"(w385) -> ()
      n437 = local write "LC_Cue2_PostR_Tdelay"(w384) -> ()
      n438 = local write "LC_Cue2_PostR_delayOpt"(w387) -> ()
      n439 = local write "LC_Cue2_PostR_Count"(w383) -> ()
      n440 = Index Array(array=w378, index #1=w557, index #2=w556, index #3=w555, index #4=w554, index #5=w553, index #6=w552, index #7=w551, index #8=w550, index #9=w549, index #10=w548, index #11=w547, index #12=w546, index #13=w545, index #14=w544, index #15=w543) -> (element #1=w539:u16, element #2=w538:u16, element #3=w537:u16, element #4=w536:u16, element #5=w535:u16, element #6=w534:u16, element #7=w533:u16, element #8=w532:u16, element #9=w531:u16, element #10=w530:u16, element #11=w529:u16, element #12=w528:u16, element #13=w527:u16, element #14=w526:u16, element #15=w525:u16)
      n441 = Not Equal To 0?(x=w512) -> (x != 0?=w514:bool)
      n442 = Not Equal To 0?(x=w507) -> (x != 0?=w513:bool)
      n443 = Not Equal To 0?(x=w539) -> (x != 0?=w542:bool)
      n444 = Not Equal To 0?(x=w534) -> (x != 0?=w541:bool)
      n445 = Not Equal To 0?(x=w529) -> (x != 0?=w540:bool)
      n446 = Index Array(array=w378, index #1=w382, index #2=w381, index #3=w376, index #4=w375, index #5=w372, index #6=w371, index #7=w370, index #8=w369, index #9=w368, index #10=w367) -> (element #1=w380:u16, element #2=w379:u16, element #3=w374:u16, element #4=w373:u16, element #5=w366:u16, element #6=w365:u16, element #7=w364:u16, element #8=w363:u16, element #9=w362:u16, element #10=w361:u16)
      n447 = local write "LC_Reward_OnOff"(w514) -> ()
      n448 = local write "LC_Reward_Block"(w511) -> ()
      n449 = local write "LC_Reward_Trial"(w510) -> ()
      n450 = local write "LC_Reward_Probability"(w509) -> ()
      n451 = local write "LC_Reward_Tdelay"(w508) -> ()
      n452 = local write "LC_Wrong_OnOff"(w513) -> ()
      n453 = local write "LC_Wrong_Block"(w506) -> ()
      n454 = local write "LC_Wrong_Trial"(w505) -> ()
      n455 = local write "LC_Wrong_Probability"(w504) -> ()
      n456 = local write "LC_Wrong_Tdelay"(w503) -> ()
      n457 = local write "LC_Sel_First_OnOff"(w542) -> ()
      n458 = local write "LC_Sel_First_Block"(w538) -> ()
      n459 = local write "LC_Sel_First_Probability"(w537) -> ()
      n460 = local write "LC_Sel_First_Tdelay"(w536) -> ()
      n461 = local write "LC_Sel_First_Count"(w535) -> ()
      n462 = local write "LC_Sel_PreR_OnOff"(w541) -> ()
      n463 = local write "LC_Sel_PreR_Block"(w533) -> ()
      n464 = local write "LC_Sel_PreR_Probability"(w532) -> ()
      n465 = local write "LC_Sel_PreR_Tdelay"(w531) -> ()
      n466 = local write "LC_Sel_PreR_Count"(w530) -> ()
      n467 = local write "LC_Sel_PostR_OnOff"(w540) -> ()
      n468 = local write "LC_Sel_PostR_Block"(w528) -> ()
      n469 = local write "LC_Sel_PostR_Probability"(w527) -> ()
      n470 = local write "LC_Sel_PostR_Tdelay"(w526) -> ()
      n471 = local write "LC_Sel_PostR_Count"(w525) -> ()
      n472 = local write "LC_ENL_nRew1"(w380) -> ()
      n473 = local write "LC_ENL_nRew2"(w379) -> ()
      n474 = local write "LC_ENL2_nRew1"(w374) -> ()
      n475 = local write "LC_ENL2_nRew2"(w373) -> ()
      n476 = local write "LC_Cue_nRew1"(w366) -> ()
      n477 = local write "LC_Cue_nRew2"(w365) -> ()
      n478 = local write "LC_Cue2_nRew1"(w364) -> ()
      n479 = local write "LC_Cue2_nRew2"(w363) -> ()
      n480 = local write "LC_Sel_nRew1"(w362) -> ()
      n481 = local write "LC_Sel_nRew2"(w361) -> ()
    }
  }
  "output_dataLC" <- w4
  "output_dataExp" <- w1
